vi "umgt_7thJuly2026.vi"(3 "STOP CODE":bool) -> ()   [LabVIEW 2024]
uses:
  <vilib>/DAQmx/configure/timing.llb/DAQmx Timing (Sample Clock).vi
  <vilib>/Utility/file.llb/Write Delimited Spreadsheet (string).vi
  <vilib>/Utility/file.llb/Write Delimited Spreadsheet (DBL).vi
  <vilib>/Analysis/NI_AALBase.lvlib
  <vilib>/Analysis/baseanly.llb/Mean (DBL).vi
  <vilib>/DAQmx/create/channels.llb/DAQmx Create Channel (AI-Voltage-Basic).vi
  <resource>/objmgr/daqmx.rc
  <vilib>/DAQmx/create/scale.llb/DAQmx Create Scale (Linear).vi
  <vilib>/addons/control/pid/NI_PID_pid.lvlib
  f57602c8-bb00-4a83-a2e4-247f724f5f9a.vi
  4c8e6df8-a562-4faa-a768-57c69aa10fff.vi
  3436942e-08c6-4c4c-99fa-98bd9929c734.vi
  <vilib>/Utility/error.llb/DialogType.ctl
  5b89efd5-d7eb-4bb1-b1dc-7bfe89948b2c.vi
  <vilib>/KNF LAB/Driver S/Lvlib/SIMLAB_driver_lvclass/SIMLAB_driver.lvclass
  Combustor Setup LabVIEW/Comb set up 1500W transfer from C drive/Combustor Setup LabVIEW/Bronkhorst FLOW-BUS/Bronkhorst FLOW-BUS.lvlib
  <vilib>/DAQmx/write.llb/DAQmx Write (Counter Time 1Chan 1Samp).vi
  <vilib>/DAQmx/configure/timing.llb/DAQmx Timing (Implicit).vi
  <vilib>/DAQmx/create/channels.llb/DAQmx Create Channel (CO-Pulse Generation-Time).vi
  <vilib>/DAQmx/read.llb/DAQmx Read (Analog 1D DBL NChan 1Samp).vi
  <vilib>/addons/control/pid/pid.llb/PID Advanced (DBL).vi
  <vilib>/DAQmx/read.llb/DAQmx Read (Analog 1D Wfm NChan NSamp Duration).vi
  Combustor Setup LabVIEW/Comb set up 1500W transfer from C drive/Combustor Setup LabVIEW/Bronkhorst FLOW-BUS/Public/Data/Measure/Read Measure (Direct).vi
  Combustor Setup LabVIEW/Comb set up 1500W transfer from C drive/Combustor Setup LabVIEW/Bronkhorst FLOW-BUS/Public/Data/Setpoint/Read Setpoint (Direct).vi
  <vilib>/DAQmx/read.llb/DAQmx Read (Analog 2D DBL NChan NSamp).vi
  <vilib>/KNF LAB/Driver S/Lvlib/SIMLAB_driver_lvclass/PumpAddress.ctl
  <vilib>/KNF LAB/Driver S/Lvlib/SIMLAB_driver_lvclass/InitParamCluster.ctl
  <vilib>/KNF LAB/Driver S/Lvlib/SIMLAB_driver_lvclass/PumpMode.ctl
panel:
  out "FlowRate(µL/min) out 2":i32 caption="Flow Rate (µL/min)"
  in  "Required Eq Ratio Kero":dbl min=0.0 max=1.5 step=0.01 format="%#_6f"
  out "total fuel flow":dbl
  out "p+k":dbl
  out "Bronkhorst Flow rate":dbl(graph)
  out "KNF Pump flow rate":dbl(graph)
  out "Dispensed Volume Bronkhorst":dbl(graph)
  out "Dispensed Volume KNF Pump":i32(graph)
  out "Bronkhorst Fuel Capacity Unit":string
  out "Bronkhorst Fuel Setpoint":sgl caption="Setpoint Direct"
  in  "stop 2":bool
  out "Time passed (s)":dbl
  in  "save file":bool
  out "current time":timestamp
  out "Bronkhorst Fuel Flow [g/s]":dbl format="%#_4g"
  in  "Bronkhorst Fuel [g/s]":dbl min=0.0 max=2.0 step=0.01 format="%#_4g"
  in  "GetActualVolume":bool
  out "ActualVolume(µL)":i32 caption="Actual Volume (µL)"
  in  "GetActualTime":bool
  out "Actual Time":dbl format="%<%H:%M:%S%2u>t"
  in  "GetDispenseTime":bool
  out "Dispense Time out":dbl caption="Dispense Time" format="%<%H:%M:%S%2u>t"
  in  "SetDispenseTime":bool
  in  "Dispense Time in":dbl=36000.0 caption="Dispense Time" min=1.0 max=359999.0 step=0.01 format="%<%H:%M:%S%2u>t"
  in  "GetDispenseVolume":bool
  out "DispenseVolume(µL) out":i32 caption="Dispense Volume (µL)"
  in  "SetDispenseVolume":bool
  in  "DispenseVolume(µL) in":i32 caption="Dispense Volume (µL)"
  in  "GetMode":bool
  out "Mode out":T1 caption="Mode"
  in  "GetFlowRate":bool
  out "FlowRate(µL/min) out":i32 caption="Flow Rate (µL/min)"
  in  "SetFlowRate":bool
  in  "FlowRate(µL/min) in":i32 caption="Flow Rate (µL/min)"
  in  "SetMode":bool
  in  "Mode in":T1 caption="Mode"
  in  "PrimeDrain":bool
  in  "Stop":bool
  in  "Start":bool
  in  "Pause 2":bool
  in  "Reset":bool
  in  "Close":bool
  in  "Init":bool
  in  "InitParam":T2={"VISA resource name"="COM9", "Address"=0, "UnusedLRC"=FALSE, "AckActive"=TRUE} {"Address" items=["0", "1", "2", "3", "4", "5", "6", "7", "8", "9", "10", "11", "12", "13", "14", "15", "16", "17", "18", "19", "20", "21", "22", "23", "24", "25", "26", "27", "28", "29", "30", "31", "32", "33", "34", "35", "36", "37", "38", "39", "40", "41", "42", "43", "44", "45", "46", "47", "48", "49", "50", "51", "52", "53", "54", "55", "56", "57", "58", "59", "60", "61", "62", "63", "64", "65", "66", "67", "68", "69", "70", "71", "72", "73", "74", "75", "76", "77", "78", "79", "80", "81", "82", "83", "84", "85", "86", "87", "88", "89", "90", "91", "92", "93", "94", "95", "96", "97", "98", "99"]}
  out "PumpVersion":string caption="Pump Version"
  out "FirmwareVersion":string caption="Firmware Version"
  out "error":errorcluster
  out "Status":string
  out "Near Glow plug Temperature [K]":dbl
  out "Volume units 2":bool
  in  "Volume 2":dbl=40.0 format="%.2f"
  in  "Initial Direction 2":u16(ring) items=["Infuse", "Withdraw"]
  in  "Syringe Inside Diameter (19.58 mm default)\n>14.00 mm : Volume units are mL\n<14.00 mm : Volume units are µL":dbl=28.0 min=0.1 max=50.0 step=0.01 format="%#_4g"
  in  "Pump Address (0) 2":i32 format="%0#.0f"
  in  "Baud Rate (19200) 2":u32(ring)=19200 items=["19200"=19200, "9600"=9600, "2400"=2400, "1200"=1200, "300"=300]
  in  "VISA resource name 2":refnum<visa-resource-name>="COM12"
  in  "Flow rate   2":dbl=6.0 min=0.0 max=6.0 step=0.05 format="%.3f"
  in  "Units 2":i32(ring)=2 items=["microlitters per minute (µL/min)", "microlitters per hour (µL/hr)", "milliliters per minute (mL/min)", "milliliters per hour (mL/hr)"]
  out "error out 2":errorcluster
  out "Tank 4":dbl(slide)
  out "Tank 3":dbl(slide)
  out "x+y 2":i32
  in  "RUN 2":bool
  in  "PAUSE 3":bool
  in  "PAUSE 4":bool
  out "Status 2":T4
  out "Volume Dispense 2":string
  out "Overall Eq Ratio":dbl=1.0
  in  "PID CONTROL":bool
  in  "PID SETP":dbl(slide)=20000.0 caption="speed" min=20000.0 max=200000.0 step=1000.0 scale=0.0..200000.0 scale format="%#_6p"
  in  "PID gains":T5={"proportional gain (Kc)"=0.00045, "integral time (Ti, min)"=0.15, "derivative time (Td, min)"=0.0} {"derivative time (Td, min)" format="%#.6f"; "integral time (Ti, min)" format="%#.5f"; "proportional gain (Kc)" format="%#.6f"}
  in  "Engine Type":bool=TRUE caption="1500 W"
  out "Battery %":u16 format="%_2f"
  out "error out":errorcluster
  out "full":dbl
  out "LT":dbl
  out "HT":dbl
  in  "Time to wait [ms]":u32=100
  out "DC Power [W]":dbl format="%#.1f"
  out "DC Current [A]":dbl format="%#.2f"
  out "DC Voltage [V]":dbl format="%#.2f"
  out "Ramp time":dbl format="%#.1f"
  in  "Max\nRPM":dbl=1e-05 min=1e-05 max=500000.0 step=1.0 format="%#.0f"
  in  "Ramp Up":bool
  in  "Pause":bool
  in  "Ramp Down":bool
  in  "Ramp\nRate [% sec]":dbl=0.33 min=0.0 max=1000.0 step=1.0 format="%#.2f"
  in  "STOP MOTOR":bool
  out "Shaft Speed [RPM]":dbl format="%#.0f"
  out "Atmospheric Pressure":dbl
  out "Bias Voltage":dbl
  in  "Stop - Actual":bool
  in  "Fuel Shut Off":bool
  in  "Track Fuel Flow Rate":bool
  out "Range Exceeded":bool
  out "Error Present":bool
  out "Error Text":string
  in  "Propane Flow Rate Setpoint":dbl min=0.0 max=0.3 step=0.01 format="%#_3g"
  out "Measurement Data":T6
  in  "COM Port Settings":T7={"Unit ID"="A", "Baud Rate"=enum."19200", "VISA Sesssion In"="COM13"}
  out "Bearing Temperature [degC]":dbl
  out "Generator Power":i16(graph)
  out "RPM":i32(graph)
  out "Pressure Ratio":dbl(graph)
  out "Coil Temperature":dbl(graph)
  out "Required Propane Fuel Flow Rate":dbl
  out "Equivalence Ratio propane":dbl
  in  "Required Eq Ratio Propane":dbl=0.6 min=0.0 max=1.6 step=0.1
  out "Elapsed Time":dbl
  out "Propane Fuel Flow Rate [g/s]":dbl
  out "Air Flow Rate [g/s]":dbl
  in  "Record":bool
  out "Turbine Inlet Temperature [K]":dbl
  out "Generator Coil Temperature [degC]":dbl
  out "Compressor Outlet Pressure [Pa]":dbl
  out "Inlet Pressure Delta [Pa]":dbl
  in  "Voltages":tag="cDAQ9185-1F541AEMod2/ai1, cDAQ9185-1F541AEMod2/ai5,cDAQ9185-1F541AEMod2/ai22"
  in  "Throttle %":dbl(slide)=0.001 caption="speed" min=0.001 max=100.0 step=0.1 scale=0.0..100.0
  in  "Ramping mode":u8
  # "Cal 1"
  # "Cal 2"
  # "Alicat MFC"
  # "Syringe Pump"
  # "KNF Fuel Pump"
  # "Bronkhorst Flow Controller"
  # "Totalizer Timer"
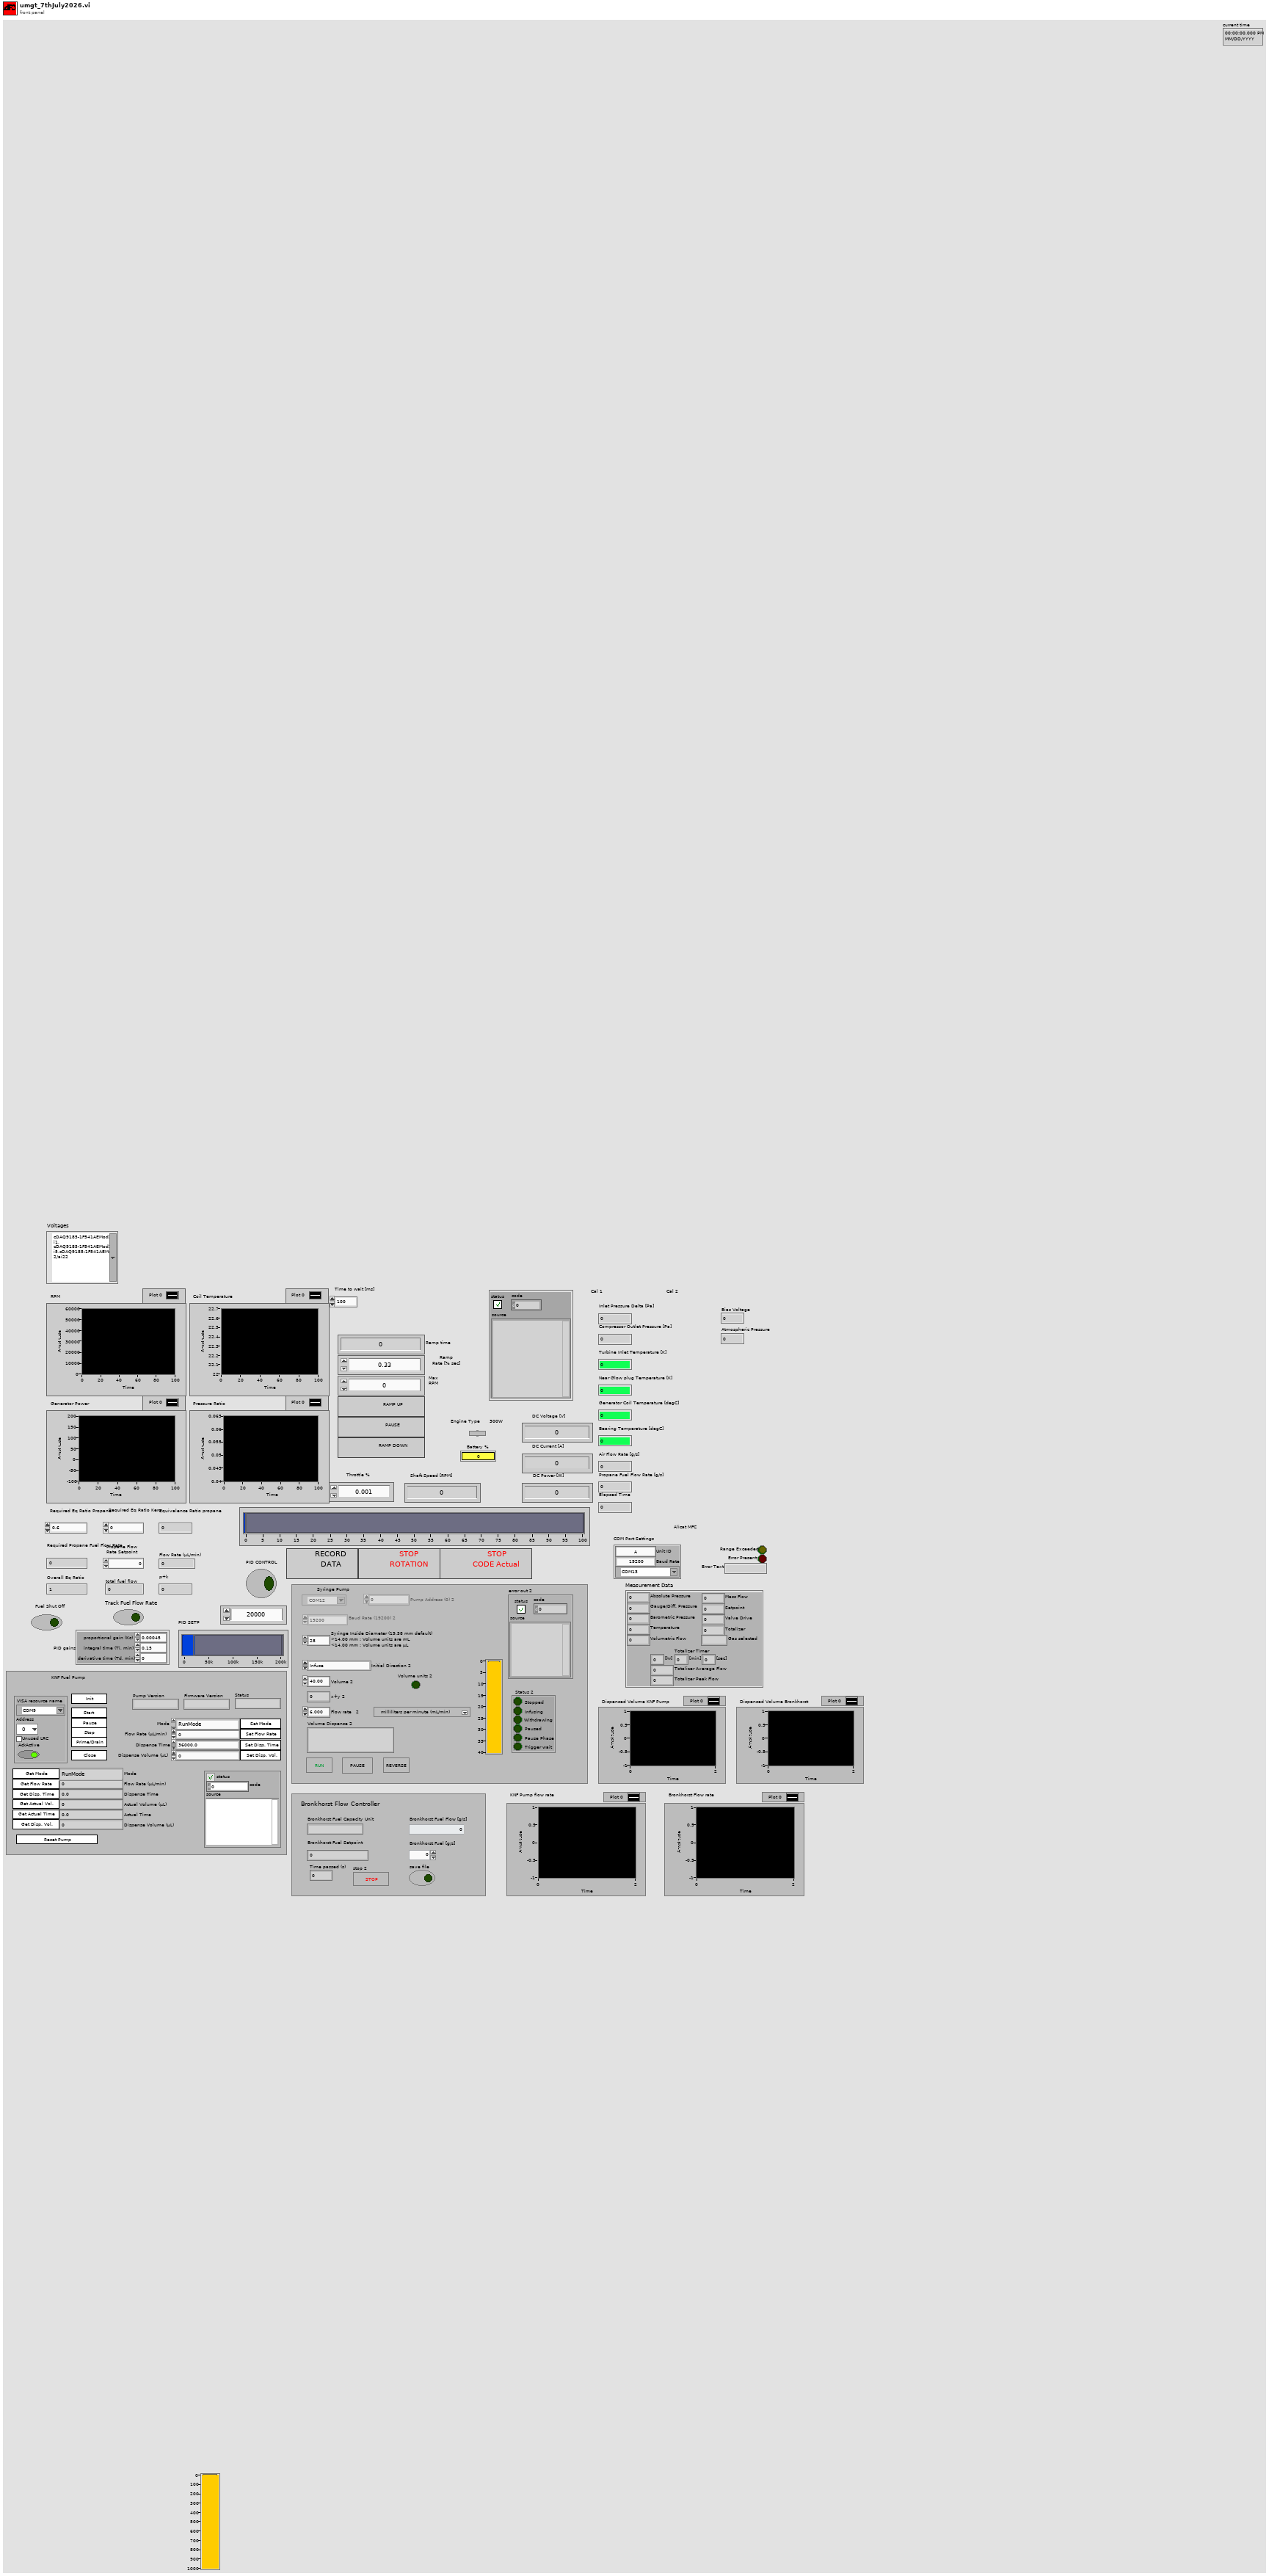
[diagram p1: front panel]
types:
  T1 = typedef "SIMLAB_driver.lvlib/SIMLAB_driver.lvclass/PumpMode.ctl" = enum16{"RunMode", "DispenseMode (mL)", "DispenseMode (mL/min)"}
  T2 = typedef "SIMLAB_driver.lvlib/SIMLAB_driver.lvclass/InitParamCluster.ctl" = cluster{"VISA resource name":refnum<visa-resource-name>, "Address":T3, "UnusedLRC":bool, "AckActive":bool}
  T3 = typedef "SIMLAB_driver.lvlib/SIMLAB_driver.lvclass/PumpAddress.ctl" = u8
  T4 = cluster{"Stopped":bool, "Infusing":bool, "Withdrawing":bool, "Paused":bool, "Pause Phase":bool, "Trigger wait":bool}
  T5 = cluster{"proportional gain (Kc)":dbl, "integral time (Ti, min)":dbl, "derivative time (Td, min)":dbl}
  T6 = cluster{"Absolute Pressure":dbl, "Gauge/Diff. Pressure":dbl, "Barometric Pressure":dbl, "Temperature":dbl, "Volumetric Flow":dbl, "Mass Flow":dbl, "Setpoint":dbl, "Valve Drive":dbl, "Totalizer":dbl, "[hr]":dbl, "[min]":dbl, "[sec]":dbl, "Totalizer Average Flow":dbl, "Totalizer Peak Flow":dbl, "Gas selected":string}
  T7 = cluster{"Unit ID":string, "Baud Rate":enum8{"2400", "9600", "19200", "38400", "57600", "115200", "Unknown"}, "VISA Sesssion In":refnum<visa-resource-name>}
  T8 = enum32{"BUS/RS232", "Analog input", "FLOW-BUS slave", "Valve close", "Controller idle", "Testing mode", "Tuning mode", "Setpoint 100%", "Valve fully open", "Calibration mode", "Analog slave", "Keyboard or FLOW-BUS setpoint", "Setpoint 0%", "FLOW-BUS analog slave", "(FPP) Range select mode", "(FPP) Manual start sensor select, automatic end sensor", "(FPP) Automatic start sensor select, manual end sensor", "(FPP) Automatic start and end sensor", "RS232 Setpoint", "RS232 broadcast mode", "Valve stearing (valve = setpoint)", "Analog valve stearing (valve = analog setpoint)", "Valve safe state"}
  T9 = typedef "DialogType.ctl" = u16
  T10 = cluster{"0=off\n1=on":u16, "Numbers of beeps\n0=continuously":dbl}
  T11 = enum8{"Enabled", "Disabled", "Disabled and Grayed Out"}
  T12 = cluster{"Absolute Pressure":bool, "Gauge/Diff. Pressure":bool, "Barometric Pressure":bool, "Temperature":bool, "Volumetric":bool, "Mass":bool, "Setpoint":bool, "Valve Drive":bool, "Totalizer":bool, "Totalizer Timer":bool, "Totalizer Average Flow":bool, "Totalizer Peak Flow":bool, "Gas Selected":bool, "Tot. Timer Format":u16}
  T13 = cluster{"Controller Full Scale":dbl, "Controller Select":u16, "Control Range":enum16{"Normal", "Inverted", "Bidirectional", "Unknown"}}
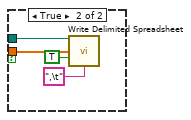
[diagram p4: hidden frame]
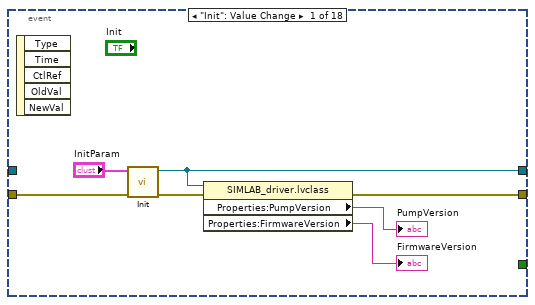
[diagram p5: hidden frame]
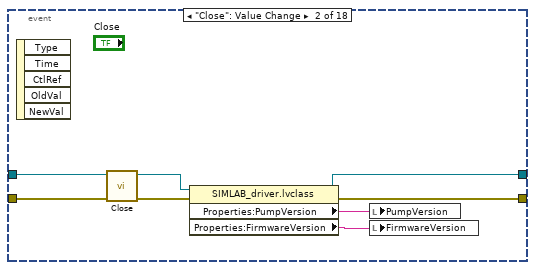
[diagram p6: hidden frame]
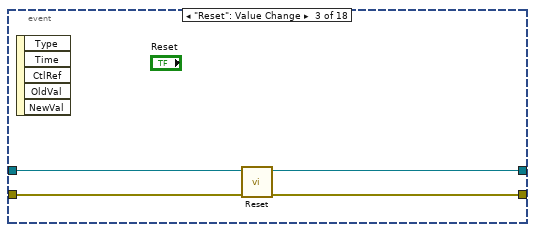
[diagram p7: hidden frame]
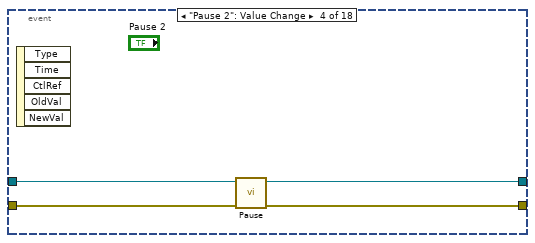
[diagram p8: hidden frame]
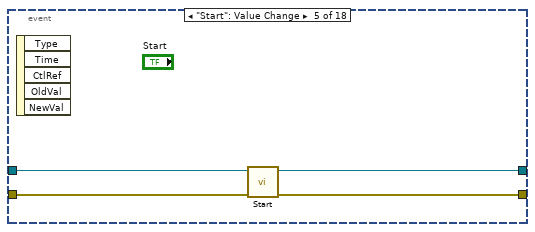
[diagram p9: hidden frame]
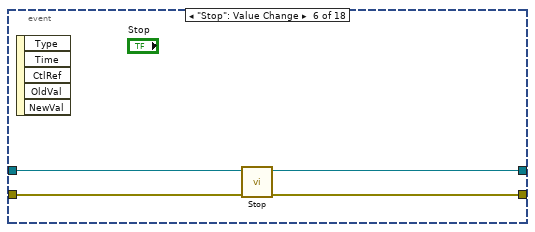
[diagram p10: hidden frame]
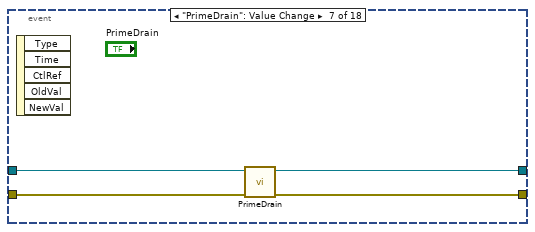
[diagram p11: hidden frame]
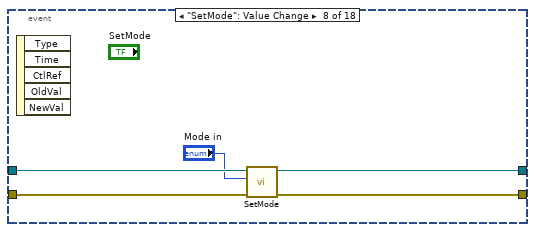
[diagram p12: hidden frame]
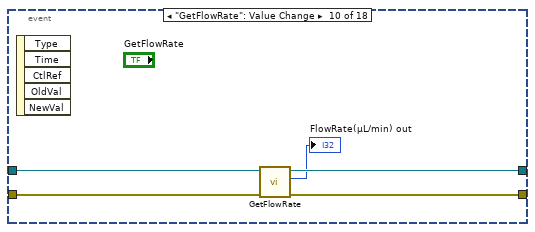
[diagram p13: hidden frame]
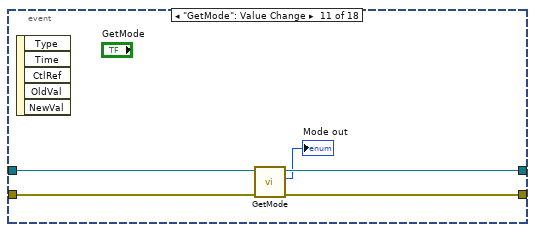
[diagram p14: hidden frame]
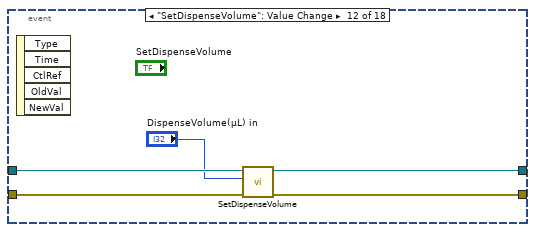
[diagram p15: hidden frame]
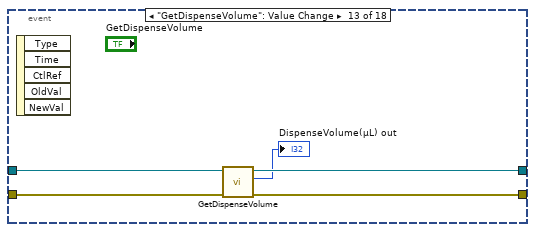
[diagram p16: hidden frame]
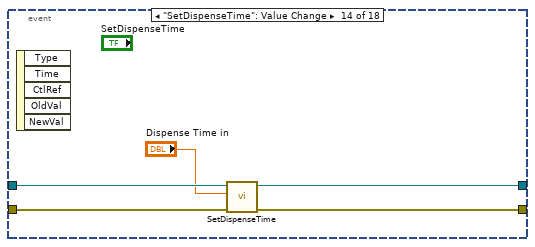
[diagram p17: hidden frame]
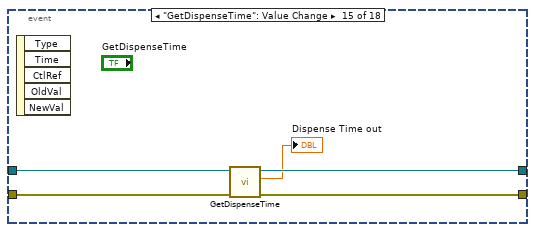
[diagram p18: hidden frame]
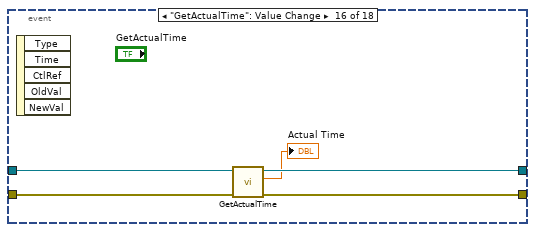
[diagram p19: hidden frame]
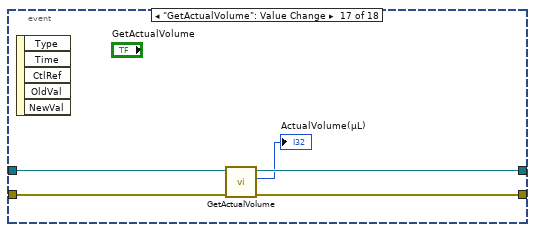
[diagram p20: hidden frame]
diagram:
  w25 = u8 3  # Node (3)
  w33 = u32 38400 items=["9600"=9600, "19200"=19200, "38400"=38400, "57600"=57600, "115200"=115200, "230400"=230400, "460800"=460800] ("Baud Rate (38400)")
  w34 = refnum<visa-resource-name> "COM5"  # VISA resource name
  w63 = T9 1 items=["no dialog", "OK message", "continue or stop message", "OK message + warnings", "continue/stop + warnings"] ("type of dialog (OK msg:1)")
  w81 = u16 0 items=["Off", "On"] ("0 = Disabled")
  # "Close the VISA session"
  # "Initialize the Com port"
  n1 = flat-sequence {
    tunnel: [w175] -> w104
    tunnel: [w174] -> w103
    tunnel: [w156] -> w102
    tunnel: [w155] -> w101
    tunnel: w104 -> [w263]
    tunnel: w103 -> [w262]
    tunnel: w102 -> [w261]
    tunnel: w101 -> [w260]
    frame #0 {
      w173 = i32[] [] ("History Data")
      n2 = Get Date/Time In Seconds() -> (seconds since 1Jan1904=w190:timestamp)
      n3 = Format Date/Time String(time format string (%c)="%y%m%d_%H_%M_%S", seconds (now)=w190) -> (date/time string=w188:string)  [unwired: 1 in]
      n4 = Concatenate Strings("D:\\UMGT Data\\Logs\\UMGT_Gen2_300W_1500W_Test_", w188, ".csv") -> (w186:string)
      n5 = Get Date/Time In Seconds() -> (seconds since 1Jan1904=w158:timestamp)
      n6 = Format Date/Time String(time format string (%c)="%y%m%d_%H_%M_%S", seconds (now)=w158) -> (date/time string=w160:string)  [unwired: 1 in]
      n7 = Concatenate Strings("D:\\UMGT Data\\Logs\\UMGT_300W_1500W_AutoLog_", w160, ".csv") -> (w162:string)
      n8 = property on="RPM" class="WFChart (strict)"("History Data"=w173) -> ()  [unwired: 2 in, 2 out]
      n9 = property on="Generator Power" class="WFChart (strict)"("History Data"=w173) -> ()  [unwired: 2 in, 2 out]
      n10 = property on="Pressure Ratio" class="WFChart (strict)"("History Data"=w173) -> ()  [unwired: 2 in, 2 out]
      n11 = property on="Coil Temperature" class="WFChart (strict)"("History Data"=w173) -> ()  [unwired: 2 in, 2 out]
      n12 = Build Array("Time [s]", "Air Flow Rate [g/s]", "Propane Fuel Flow Rate [g/s]", "Compressor Outlet Pressure [Pa]", "Coil Temperature [degC]", "Turbine Inlet Temperature [K]", "Bearing Temperature [degC]", "Controller Output Power [W]", "Shaft Speed [RPM]", "Equivalence Ratio", "Throttle %" ("element"), "Pressure Ratio" ("element"), "Overall Eq ratio" ("element"), "Inlet Pressure delta (Pa)" ("element"), "Near Glow plug Temperature (K)" ("element"), "Battery %" ("element"), "Syringe pump infuse volume" ("element"), "Syringe pump flow rate" ("element"), "KNF pump flow rate in (uL/min)" ("element"), "KNF pump flow rate out (uL/min)" ("element"), "KNF pump Dispense volume in (uL)" ("element"), "KNF pump Dispense volume out (uL)" ("element"), "KNF pump Dispense time in " ("element"), "KNF pump Dispense time out " ("element"), "Bronkhorst Fuel flow actual (g/s)" ("element"), "Bronkhorst fuel (g/s)" ("element"), "Bronkhorst Fuel set point (g/s)" ("element"), "DC Current (A)" ("element"), "DC Voltage (V)" ("element"), "Required Eq Ratio Kerosene" ("element"), "Kerosene fuel flow rate KNF (ul/min) 2 " ("element")) -> (w172:string[])
      n13 = String To Path(string=w186) -> (path=w185:path)
      n14 = String To Path(string=w162) -> (path=w163:path)
      n15 = call-poly <vilib>:"Write Delimited Spreadsheet.vi"("file path (dialog if empty)"=w163, "1D data"=w172, "delimiter (\\t)"="," ("delimiter (\\t)")) -> ("new file path (Not A Path if cancelled)"=w156:path, "error out"=w155:errorcluster)  [unwired: 11 in]
      n16 = Build Array("Time [s]", "Air Flow Rate [g/s]", "Propane Fuel Flow Rate [g/s]", "Compressor Outlet Pressure [Pa]", "Coil Temperature [degC]", "Turbine Inlet Temperature [K]", "Bearing Temperature [degC]", "Controller Output Power [W]", "Shaft Speed [RPM]", "Equivalence Ratio", "Throttle %" ("element"), "Pressure Ratio" ("element"), "Overall Eq ratio" ("element"), "Inlet Pressure Delta (Pa)" ("element"), "Near Glow plug Temperature (K)" ("element"), "Battery %" ("element"), "Syringe pump infuse volume" ("element"), "Syringe pump flow rate" ("element"), "KNF pump flow rate in (uL/min)" ("element"), "KNF pump flow rate out (uL/min)" ("element"), "KNF pump Dispense volume in (uL)" ("element"), "KNF pump Dispense volume out (uL)" ("element"), "KNF pump Dispense time in " ("element"), "KNF pump Dispense time out " ("element"), "Bronkhorst Fuel flow actual (g/s)" ("element"), "Bronkhorst fuel (g/s)" ("element"), "Bronkhorst Fuel set point (g/s)" ("element"), "DC Current (A)" ("element"), "DC Voltage (V)" ("element"), "Required Eq Ratio Kerosene" ("element"), "Kerosene fuel flow rate KNF (ul/min) 2 " ("element")) -> (w176:string[])
      n17 = call-poly <vilib>:"Write Delimited Spreadsheet.vi"("file path (dialog if empty)"=w185, "1D data"=w176, "delimiter (\\t)"="," ("delimiter (\\t)")) -> ("new file path (Not A Path if cancelled)"=w175:path, "error out"=w174:errorcluster)  [unwired: 11 in]
      "Bias Voltage" <- 0.0 ("Bias Voltage")
      "Atmospheric Pressure" <- 98600.0 ("Atmospheric Pressure")
    }
    frame #1 {
      w223 = 10106 items=["Default"=-1, "RSE"=10083, "NRSE"=10078, "Differential"=10106, "Pseudodifferential"=12529] ("input terminal configuration")
      w220 = 10123 items=["Finite Samples"=10178, "Continuous Samples"=10123, "Hardware Timed Single Point"=12522] ("sample mode")
      w214 = 10348 items=["Volts"=10348, "Amps"=10342, "Deg F"=10144, "Deg C"=10143, "Deg R"=10145, "Kelvins"=10325, "Strain"=10299, "Ohms"=10384, "Hz"=10373, "Seconds"=10364, "Meters"=10219, "Inches"=10379, "Degrees"=10146, "Radians"=10273, "Ticks"=10304, "g"=10186, "m/s^2"=12470, "m/s"=15959, "in/s"=15960, "Pascals"=10081, "Newtons"=15875, "Pounds"=15876, "kgf"=15877, "psi"=15879, "bar"=15880, "Nm"=15881, "oz-in"=15882, "lb-in"=15883, "lb-ft"=15884, "Volts/Volt"=15896, "mVolts/Volt"=15897, "pCoulombs"=16103, "Coulombs"=16102, "From TEDS"=12516] ("pre-scaled units")
      w206 = 10106 items=["Default"=-1, "RSE"=10083, "NRSE"=10078, "Differential"=10106, "Pseudodifferential"=12529] ("input terminal configuration")
      w200 = 10106 items=["Default"=-1, "RSE"=10083, "NRSE"=10078, "Differential"=10106, "Pseudodifferential"=12529] ("input terminal configuration")
      w210 = 10348 items=["Volts"=10348, "Amps"=10342, "Deg F"=10144, "Deg C"=10143, "Deg R"=10145, "Kelvins"=10325, "Strain"=10299, "Ohms"=10384, "Hz"=10373, "Seconds"=10364, "Meters"=10219, "Inches"=10379, "Degrees"=10146, "Radians"=10273, "Ticks"=10304, "g"=10186, "m/s^2"=12470, "m/s"=15959, "in/s"=15960, "Pascals"=10081, "Newtons"=15875, "Pounds"=15876, "kgf"=15877, "psi"=15879, "bar"=15880, "Nm"=15881, "oz-in"=15882, "lb-in"=15883, "lb-ft"=15884, "Volts/Volt"=15896, "mVolts/Volt"=15897, "pCoulombs"=16103, "Coulombs"=16102, "From TEDS"=12516] ("pre-scaled units")
      w203 = 10065 items=["Volts"=10348, "From Custom Scale"=10065] ("units")
      w197 = 10065 items=["Volts"=10348, "From Custom Scale"=10065] ("units")
      w192 = 10214 items=["High"=10192, "Low"=10214] ("idle state")
      w195 = 10123 items=["Finite Samples"=10178, "Continuous Samples"=10123, "Hardware Timed Single Point"=12522] ("sample mode")
      w285 = 10123 items=["Finite Samples"=10178, "Continuous Samples"=10123, "Hardware Timed Single Point"=12522] ("sample mode")
      w286 = 10123 items=["Finite Samples"=10178, "Continuous Samples"=10123, "Hardware Timed Single Point"=12522] ("sample mode")
      w291 = 10106 items=["Default"=-1, "RSE"=10083, "NRSE"=10078, "Differential"=10106, "Pseudodifferential"=12529] ("input terminal configuration")
      n18 = call-poly <vilib>:"DAQmx Create Scale.vi"("name"="SSA100-1", "slope"=80.0 ("x"), "pre-scaled units"=w210, "scaled units"="Amps") -> ("scale out"=w241:tag)  [unwired: 10 in, 1 out]
      n19 = call <vilib>:"Clear Errors.vi"() -> ("error out"=w239:errorcluster)  [unwired: 6 in, 1 out]
      n20 = call-poly <vilib>:"DAQmx Create Scale.vi"("name"="Divider", "slope"=11.0, "y-intercept"=0.0, "pre-scaled units"=w214, "scaled units"="Volts") -> ("scale out"=w240:tag)  [unwired: 9 in, 1 out]
      n21 = call-poly <vilib>:"DAQmx Create Virtual Channel.vi"("maximum value"=10.0, "minimum value"=0.0, "input terminal configuration"=w291, "physical channels"="Voltages") -> ("task out"=w288:refnum<k21>, "error out"=w287:errorcluster)  [unwired: 10 in]
      n22 = call-poly <vilib>:"DAQmx Create Virtual Channel.vi"("maximum value"=800.0, "minimum value"=-800.0, "input terminal configuration"=w200, "physical channels"=tag "cDAQ9185-1F541AEMod4/ai0", "name to assign"="MotorCurrent", "units"=w197, "error in"=w239, "custom scale name"=w241) -> ("task out"=w242:refnum<k21>, "error out"=w243:errorcluster)  [unwired: 6 in]
      n23 = call-poly <vilib>:"DAQmx Timing.vi"("task/channels in"=refnum<k21> "Near Glow Plug Temperature, Coil Temperature, Turbine Inlet Temperature, Bearing Temperature", "sample mode"=w285, "samples per channel"=1, "rate"=5.0) -> ("task out"=w278:refnum<k21>, "error out"=w277:errorcluster)  [unwired: 10 in]
      n24 = call-poly <vilib>:"DAQmx Create Virtual Channel.vi"("task in"=w242, "maximum value"=110.0, "minimum value"=-110.0, "input terminal configuration"=w206, "physical channels"=tag "cDAQ9185-1F541AEMod4/ai1", "name to assign"="MotorVoltage", "units"=w203, "error in"=w243, "custom scale name"=w240) -> ("task out"=w244:refnum<k21>, "error out"=w245:errorcluster)  [unwired: 5 in]
      n25 = call <vilib>:"Clear Errors.vi"() -> ("error out"=w238:errorcluster)  [unwired: 6 in, 1 out]
      n26 = call-poly <vilib>:"DAQmx Create Virtual Channel.vi"("task in"=w244, "maximum value"=5.0, "minimum value"=-5.0, "input terminal configuration"=w223, "physical channels"=tag "cDAQ9185-1F541AEMod4/ai2" ("counter"), "name to assign"="MotorSpeed", "error in"=w245) -> ("task out"=w246:refnum<k21>, "error out"=w247:errorcluster)  [unwired: 7 in]
      n27 = call-poly <vilib>:"DAQmx Create Virtual Channel.vi"("counter"=tag "cDAQ9185-1F541AEMod3/ctr0", "name to assign"="MotorPulse", "error in"=w238, "idle state"=w192) -> ("task out"=w234:refnum<k21>, "error out"=w235:errorcluster)  [unwired: 10 in]
      n28 = call-poly <vilib>:"DAQmx Timing.vi"("task/channels in"=w288, "sample mode"=w286, "samples per channel"=1, "rate"=150.0, "error in"=w287) -> ("task out"=w280:refnum<k21>, "error out"=w279:errorcluster)  [unwired: 9 in]
      n29 = property class="DAQmx Channel"(reference=w234, error in=w235, "CO.Pulse.Term"=tag "/cDAQ9185-1F541AEMod3/PFI0") -> (reference out=w236:refnum<k21>, error out=w237:errorcluster)
      n30 = call-poly <vilib>:"DAQmx Timing.vi"("task/channels in"=w246, "sample mode"=w220, "rate"=10000.0, "source"=tag "OnboardClock", "error in"=w247) -> ("task out"=w254:refnum<k21>, "error out"=w255:errorcluster)  [unwired: 9 in]
      n31 = call <vilib>:"DAQmx Start Task.vi"("task/channels in"=w278, "error in"=w277) -> ("task out"=w274:refnum<k21>, "error out"=w273:errorcluster)  [unwired: 12 in]
      n32 = call <vilib>:"DAQmx Start Task.vi"("task/channels in"=w280, "error in"=w279) -> ("task out"=w276:refnum<k21>, "error out"=w275:errorcluster)  [unwired: 12 in]
      n33 = call-poly <vilib>:"DAQmx Timing.vi"("task/channels in"=w236, "sample mode"=w195, "error in"=w237) -> ("task out"=w229:refnum<k21>, "error out"=w228:errorcluster)  [unwired: 11 in]
      n34 = call <vilib>:"DAQmx Start Task.vi"("task/channels in"=w254, "error in"=w255) -> ("task out"=w252:refnum<k21>, "error out"=w253:errorcluster)  [unwired: 12 in]
      n35 = call <vilib>:"High Resolution Relative Seconds.vi"() -> ("relative seconds"=w264:dbl)
      n36 = call <vilib>:"DAQmx Start Task.vi"("task/channels in"=w229, "error in"=w228) -> ("task out"=w230:refnum<k21>, "error out"=w231:errorcluster)  [unwired: 12 in]
      n37 = while {
        tunnel: w276 -> [w584]
        tunnel: w275 -> [w583]
        tunnel: w274 -> [w582]
        tunnel: w273 -> [w581]
        tunnel: [w580] -> w272
        tunnel: [w579] -> w271
        tunnel: w264 -> [w571]
        tunnel: w263 -> [w570]
        tunnel: w262 -> [w569]
        tunnel: w261 -> [w559]
        tunnel: w260 -> [w557]
        tunnel: [w508] -> w257
        tunnel: [w507] -> w256
        stop <- w578 stop-if-true
        # "change mdot from 0.702 for 1500W to 0.54 for 300W"
        # "KNF pump kerosene"
        # "changed from 15.67 to 15.5"
        # "changed from 15.67 to 15.5"
        # "ml/min to g/s\n(0.84/60)"
        # "stoichiometric propane"
        # "stoichiometric kero"
        # "Propane gas"
        # "Kerosene from syringe pump"
        n38 = call-poly <vilib>:"DAQmx Read.vi"("task/channels in"=w584, "number of samples per channel"=20, "error in"=w583) -> ("task out"=w508:refnum<k21>, "data"=w561:dbl[][], "error out"=w507:errorcluster)  [unwired: 10 in]
        n39 = Index Array(array=w561, index (row)=1 ("index")) -> (element=w547:dbl[])  [unwired: 1 in]
        n40 = Index Array(array=w561, index (row)=0 ("index")) -> (element=w548:dbl[])  [unwired: 1 in]
        n41 = call-poly <vilib>:"Mean.vi"("X"=w547) -> ("mean"=w509:dbl)  [unwired: 1 out]
        n42 = call-poly <vilib>:"Mean.vi"("X"=w548) -> ("mean"=w484:dbl)  [unwired: 1 out]
        n43 = formula code="P = 50*V;"("V"=w484) -> ("P"=w468:dbl)
        "Inlet Pressure Delta [Pa]" <- w468
        n44 = formula code="P = 16000*V;"("V"=w509) -> ("P"=w506:dbl)
        "Compressor Outlet Pressure [Pa]" <- w506
        n45 = formula code="mdot = 0.702*sqrt(Pin);"("Pin"=w468) -> ("mdot"=w566:dbl)
        "Air Flow Rate [g/s]" <- w566
        n46 = local read "Atmospheric Pressure"() -> (w513:dbl)
        n47 = local read "FlowRate(µL/min) out"() -> (w479:i32)
        n48 = local read "Measurement Data"() -> (w553:T6)
        n49 = local read "Propane Fuel Flow Rate [g/s]"() -> (w487:dbl)
        n50 = local read "Flow rate   2"() -> (w511:dbl)
        n51 = Divide(x=w506, y=w513) -> (x/y=→"Pressure Ratio":dbl)
        n52 = Multiply(x=w479, y=1.33e-05) -> (x*y=w473:dbl)
        n53 = Unbundle By Name(w553) -> ("Mass Flow"=w552:dbl)
        "Propane Fuel Flow Rate [g/s]" <- w552
        n54 = Multiply(x=w511, y=0.014) -> (x*y=w490:dbl)
        n55 = Multiply(x=15.0, y=w490) -> (x*y=w489:dbl)
        n56 = Multiply(x=15.5, y=w487) -> (x*y=w475:dbl)
        n57 = Multiply(x=15.0, y=w473) -> (x*y=w476:dbl)
        n58 = Divide(x=w566, y=w552) -> (x/y=w568:dbl)
        n59 = Multiply(x="Required Eq Ratio Propane", y=w566) -> (x*y=w564:dbl)
        n60 = Reciprocal(x=15.5) -> (1/x=w563:dbl)
        n61 = Add(x=w476, y=w475) -> (x+y=w471:dbl)
        n62 = Add(x=w489, y=w475) -> (x+y=w470:dbl)
        n63 = Divide(x=w568, y=15.5) -> (x/y=w551:dbl)
        n64 = Multiply(x=w564, y=w563) -> (x*y=→"Required Propane Fuel Flow Rate":dbl)
        n65 = Add(x=w471, y=w470) -> (x+y=w472:dbl)
        "total fuel flow" <- w472
        n66 = Reciprocal(x=w551) -> (1/x=→"Equivalence Ratio propane":dbl)
        n67 = local read "Air Flow Rate [g/s]"() -> (w486:dbl)
        n68 = Divide(x=w472, y=w486) -> (x/y=→"Overall Eq Ratio":dbl)
        n69 = disable-structure shown="Disabled" {
          frame Disabled {
            n70 = case shown="True" "Track Fuel Flow Rate" {
              frame False {
              }
              frame True {
                n71 = local read "Required Propane Fuel Flow Rate"() -> (w588:dbl)
                n72 = local read "Required Eq Ratio Kero"() -> (w587:dbl)
                n73 = Add(x=w588, y=w587) -> (x+y=w586:dbl)
                n74 = local write "Propane Flow Rate Setpoint"(w588) -> ()
                n75 = local write "p+k"(w586) -> ()
              }
            }
          }
          frame Enabled {
          }
        }
        n76 = case shown="True" "Fuel Shut Off" {
          frame False {
          }
          frame True {
            n77 = local write "Fuel Shut Off"(FALSE ("Fuel Shut Off")) -> ()
            n78 = local write "Propane Flow Rate Setpoint"(0.0 ("Fuel Flow Rate Setpoint")) -> ()
            n79 = property on="Stop" class="Bool (strict)"("Val(Sgnl)"=TRUE) -> ()  [unwired: 2 in, 2 out]
          }
        }
        n80 = local read "Dispensed Volume Bronkhorst"() -> (→"Dispensed Volume Bronkhorst":dbl)
        n81 = local read "FlowRate(µL/min) out"() -> (→"FlowRate(µL/min) out 2":i32)
        n82 = call "Elapsed Time"() -> ("Time has Elapsed"=w560:bool)  [unwired: 12 in, 7 out]
        n83 = local read "KNF Pump flow rate"() -> (→"KNF Pump flow rate":dbl)
        n84 = local read "DispenseVolume(µL) out"() -> (→"Dispensed Volume KNF Pump":i32)
        n85 = local read "Bronkhorst Flow rate"() -> (→"Bronkhorst Flow rate":dbl)
        n86 = call-poly <vilib>:"DAQmx Read.vi"("task/channels in"=w582, "error in"=w581) -> ("task out"=w580:refnum<k21>, "data"=w502:dbl[], "error out"=w579:errorcluster)  [unwired: 11 in]
        n87 = Index Array(array=w502, index=2) -> (element=w555:dbl)
        n88 = Index Array(array=w502, index=1) -> (element=w535:dbl)
        "Generator Coil Temperature [degC]" <- w535
        "Coil Temperature" <- w535
        n89 = Add(x=w555, y=273.15) -> (x+y=w515:dbl)
        "Turbine Inlet Temperature [K]" <- w515
        n90 = Index Array(array=w502, index=3) -> (element=w525:dbl)
        "Bearing Temperature [degC]" <- w525
        n91 = call <vilib>:"High Resolution Relative Seconds.vi"() -> ("relative seconds"=w572:dbl)
        n92 = Subtract(x=w572, y=w571) -> (x-y=w558:dbl)
        "Elapsed Time" <- w558
        n93 = Less Or Equal?(x=w535, y=90.0) -> (x <= y?=w540:bool)
        n94 = Greater Or Equal?(x=w535, y=50.0) -> (x >= y?=w539:bool)
        n95 = Greater?(x=w535, y=90.0) -> (0:w537:bool)
        n96 = Less?(x=w535, y=50.0) -> (x < y?=w543:bool)
        n97 = And(x=w540, y=w539) -> (x .and. y?=w538:bool)
        n98 = local read "STOP CODE"() -> (w578:bool)
        n99 = case shown="True" "Record" {
          tunnel: w558 -> [_ w681]
          tunnel: w570 -> [_ w675]
          tunnel: w569 -> [_ w674]
          frame False {
          }
          frame True {
            n100 = local read "Generator Coil Temperature [degC]"() -> (w677:dbl)
            n101 = local read "Near Glow plug Temperature [K]"() -> (w662:dbl)
            n102 = local read "Compressor Outlet Pressure [Pa]"() -> (w678:dbl)
            n103 = local read "Turbine Inlet Temperature [K]"() -> (w670:dbl)
            n104 = local read "Propane Fuel Flow Rate [g/s]"() -> (w679:dbl)
            n105 = local read "Bearing Temperature [degC]"() -> (w669:dbl)
            n106 = local read "DispenseVolume(µL) out"() -> (w655:i32)
            n107 = local read "Inlet Pressure Delta [Pa]"() -> (w663:dbl)
            n108 = local read "DispenseVolume(µL) in"() -> (w656:i32)
            n109 = local read "Equivalence Ratio propane"() -> (w667:dbl)
            n110 = local read "FlowRate(µL/min) out"() -> (w657:i32)
            n111 = local read "Bronkhorst Fuel Flow [g/s]"() -> (w652:dbl)
            n112 = local read "Bronkhorst Fuel Setpoint"() -> (w650:sgl)
            n113 = local read "FlowRate(µL/min) in"() -> (w658:i32)
            n114 = local read "Required Eq Ratio Kero"() -> (w647:dbl)
            n115 = local read "FlowRate(µL/min) out 2"() -> (w646:i32)
            n116 = local read "Shaft Speed [RPM]"() -> (w676:dbl)
            n117 = local read "Dispense Time out"() -> (w653:dbl)
            n118 = local read "Air Flow Rate [g/s]"() -> (w680:dbl)
            n119 = local read "Dispense Time in"() -> (w654:dbl)
            n120 = local read "Overall Eq Ratio"() -> (w664:dbl)
            n121 = local read "Bronkhorst Fuel [g/s]"() -> (w651:dbl)
            n122 = local read "Pressure Ratio"() -> (w665:dbl)
            n123 = local read "DC Power [W]"() -> (w671:dbl)
            n124 = local read "Flow rate   2"() -> (w659:dbl)
            n125 = local read "Throttle %"() -> (w666:dbl)
            n126 = local read "DC Current [A]"() -> (w649:dbl)
            n127 = local read "DC Voltage [V]"() -> (w648:dbl)
            n128 = local read "Battery %"() -> (w661:u16)
            n129 = local read "Tank 4"() -> (w660:dbl)
            n130 = Build Array(w681, w680, w679, w678, w677, w670, w669, w671, w676, w667, w666, w665, w664, w663, w662, w661, w660, w659, w658, w657, w656, w655, w654, w653, w652, w651, w650, w649, w648, w647, w646) -> (w672:dbl[])
            n131 = call-poly <vilib>:"Write Delimited Spreadsheet.vi"("file path (dialog if empty)"=w675, "1D data"=w672, "append to file? (new file:F)"=TRUE, "error in (no error)"=w674, "delimiter (\\t)"="," ("delimiter (\\t)")) -> ()  [unwired: 9 in, 2 out]
          }
        }
        n132 = case shown="True" w543 {
          frame False {
          }
          frame True {
            n133 = property on="Generator Coil Temperature [degC]" class="DigNum (strict)"("NumText.BGColor"=u32 1245013 ("Color Box")) -> ()  [unwired: 2 in, 2 out]
          }
        }
        n134 = case shown="False" w538 {
          frame False {
          }
          frame True {
            n135 = property on="Generator Coil Temperature [degC]" class="DigNum (strict)"("NumText.BGColor"=u32 16776770 ("Color Box")) -> ()  [unwired: 2 in, 2 out]
          }
        }
        n136 = case shown="False" w537 {
          frame False {
          }
          frame True {
            n137 = property on="Generator Coil Temperature [degC]" class="DigNum (strict)"("NumText.BGColor"=u32 16726826 ("Color Box")) -> ()  [unwired: 2 in, 2 out]
          }
        }
        n138 = Index Array(array=w502, index=0) -> (element=w503:dbl)
        n139 = case shown="True" w560 {
          tunnel: w558 -> [_ w645]
          tunnel: w559 -> [_ w638]
          tunnel: w557 -> [_ w637]
          frame False {
          }
          frame True {
            n140 = local read "Generator Coil Temperature [degC]"() -> (w641:dbl)
            n141 = local read "Overall Eq Ratio"() -> (w628:dbl)
            n142 = local read "Compressor Outlet Pressure [Pa]"() -> (w642:dbl)
            n143 = local read "Turbine Inlet Temperature [K]"() -> (w640:dbl)
            n144 = local read "Bearing Temperature [degC]"() -> (w633:dbl)
            n145 = local read "Near Glow plug Temperature [K]"() -> (w626:dbl)
            n146 = local read "Bronkhorst Fuel Flow [g/s]"() -> (w616:dbl)
            n147 = local read "Propane Fuel Flow Rate [g/s]"() -> (w643:dbl)
            n148 = local read "Bronkhorst Fuel Setpoint"() -> (w614:sgl)
            n149 = local read "Equivalence Ratio propane"() -> (w631:dbl)
            n150 = local read "Required Eq Ratio Kero"() -> (w611:dbl)
            n151 = local read "FlowRate(µL/min) out 2"() -> (w610:i32)
            n152 = local read "Inlet Pressure Delta [Pa]"() -> (w627:dbl)
            n153 = local read "Bronkhorst Fuel [g/s]"() -> (w615:dbl)
            n154 = local read "DispenseVolume(µL) out"() -> (w618:i32)
            n155 = local read "DC Power [W]"() -> (w634:dbl)
            n156 = local read "DispenseVolume(µL) in"() -> (w617:i32)
            n157 = local read "FlowRate(µL/min) out"() -> (w621:i32)
            n158 = local read "Pressure Ratio"() -> (w629:dbl)
            n159 = local read "Air Flow Rate [g/s]"() -> (w644:dbl)
            n160 = local read "Dispense Time out"() -> (w620:dbl)
            n161 = local read "Throttle %"() -> (w630:dbl)
            n162 = local read "FlowRate(µL/min) in"() -> (w622:i32)
            n163 = local read "Flow rate   2"() -> (w623:dbl)
            n164 = local read "Dispense Time in"() -> (w619:dbl)
            n165 = local read "Shaft Speed [RPM]"() -> (w639:dbl)
            n166 = local read "DC Current [A]"() -> (w613:dbl)
            n167 = local read "DC Voltage [V]"() -> (w612:dbl)
            n168 = local read "Battery %"() -> (w625:u16)
            n169 = local read "Tank 4"() -> (w624:dbl)
            n170 = Build Array(w645, w644, w643, w642, w641, w640, w633, w634, w639, w631, w630, w629, w628, w627, w626, w625, w624, w623, w622, w621, w617, w618, w619, w620, w616, w615, w614, w613, w612, w611, w610) -> (w635:dbl[])
            n171 = call-poly <vilib>:"Write Delimited Spreadsheet.vi"("file path (dialog if empty)"=w638, "1D data"=w635, "append to file? (new file:F)"=TRUE, "error in (no error)"=w637, "delimiter (\\t)"="," ("delimiter (\\t)")) -> ()  [unwired: 9 in, 2 out]
          }
        }
        n172 = Add(x=w503, y=273.15) -> (x+y=w497:dbl)
        "Near Glow plug Temperature [K]" <- w497
        n173 = Less Or Equal?(x=w525, y=90.0) -> (x <= y?=w530:bool)
        n174 = Greater Or Equal?(x=w525, y=50.0) -> (x >= y?=w531:bool)
        n175 = Greater?(x=w525, y=90.0) -> (0:w533:bool)
        n176 = Less?(x=w525, y=50.0) -> (x < y?=w527:bool)
        n177 = And(x=w530, y=w531) -> (x .and. y?=w532:bool)
        n178 = case shown="True" w527 {
          frame False {
          }
          frame True {
            n179 = property on="Bearing Temperature [degC]" class="DigNum (strict)"("NumText.BGColor"=u32 1245013 ("Color Box")) -> ()  [unwired: 2 in, 2 out]
          }
        }
        n180 = case shown="False" w532 {
          frame False {
          }
          frame True {
            n181 = property on="Bearing Temperature [degC]" class="DigNum (strict)"("NumText.BGColor"=u32 16776770 ("Color Box")) -> ()  [unwired: 2 in, 2 out]
          }
        }
        n182 = case shown="False" w533 {
          frame False {
          }
          frame True {
            n183 = property on="Bearing Temperature [degC]" class="DigNum (strict)"("NumText.BGColor"=u32 16726826 ("Color Box")) -> ()  [unwired: 2 in, 2 out]
          }
        }
        n184 = local read "Time to wait [ms]"() -> (w512:u32)
        n185 = Wait (ms)(milliseconds to wait=w512) -> ()  [unwired: 1 out]
        n186 = Less Or Equal?(x=w515, y=1050.0) -> (x <= y?=w520:bool)
        n187 = Greater Or Equal?(x=w515, y=500.0) -> (x >= y?=w519:bool)
        n188 = Greater?(x=w515, y=1050.0) -> (0:w517:bool)
        n189 = Less?(x=w515, y=500.0) -> (x < y?=w523:bool)
        n190 = And(x=w520, y=w519) -> (x .and. y?=w518:bool)
        n191 = case shown="True" w523 {
          frame False {
          }
          frame True {
            n192 = property on="Turbine Inlet Temperature [K]" class="DigNum (strict)"("NumText.BGColor"=u32 1245013 ("Color Box")) -> ()  [unwired: 2 in, 2 out]
          }
        }
        n193 = case shown="False" w518 {
          frame False {
          }
          frame True {
            n194 = property on="Turbine Inlet Temperature [K]" class="DigNum (strict)"("NumText.BGColor"=u32 16776770 ("Color Box")) -> ()  [unwired: 2 in, 2 out]
          }
        }
        n195 = case shown="False" w517 {
          frame False {
          }
          frame True {
            n196 = property on="Turbine Inlet Temperature [K]" class="DigNum (strict)"("NumText.BGColor"=u32 16726826 ("Color Box")) -> ()  [unwired: 2 in, 2 out]
          }
        }
        n197 = case shown="True" "Stop - Actual" {
          frame False {
          }
          frame True {
            n198 = local read "Shaft Speed [RPM]"() -> (w592:dbl)
            n199 = Less Or Equal?(x=w592, y=10000) -> (x <= y?=w593:bool)
            n200 = case shown="False" w593 {
              frame False {
                n201 = local write "Stop - Actual"(FALSE ("Stop - Actual")) -> ()
                n202 = One Button Dialog(message="Can't stop code while motor running") -> ()  [unwired: 1 in, 1 out]
              }
              frame True {
                n203 = local write "STOP CODE"(TRUE ("stop")) -> ()
              }
            }
          }
        }
        n204 = Less Or Equal?(x=w497, y=1050.0 ("x+y")) -> (x <= y?=w494:bool)
        n205 = Greater Or Equal?(x=w497, y=500.0) -> (x >= y?=w495:bool)
        n206 = Less?(x=w497, y=500.0) -> (x < y?=w501:bool)
        n207 = And(x=w494, y=w495) -> (x .and. y?=w500:bool)
        n208 = Greater?(x=w497, y=1050.0) -> (0:w492:bool)
        n209 = case shown="True" w501 {
          frame False {
          }
          frame True {
            n210 = property on="Near Glow plug Temperature [K]" class="DigNum (strict)"("NumText.BGColor"=u32 1245013 ("Color Box")) -> ()  [unwired: 2 in, 2 out]
          }
        }
        n211 = case shown="False" w500 {
          frame False {
          }
          frame True {
            n212 = property on="Near Glow plug Temperature [K]" class="DigNum (strict)"("NumText.BGColor"=u32 16776770 ("Color Box")) -> ()  [unwired: 2 in, 2 out]
          }
        }
        n213 = case shown="False" w492 {
          frame False {
          }
          frame True {
            n214 = property on="Near Glow plug Temperature [K]" class="DigNum (strict)"("NumText.BGColor"=u32 16726826 ("Color Box")) -> ()  [unwired: 2 in, 2 out]
          }
        }
      }
      n215 = while {
        stop <- w386 stop-if-true
        w382 = u32 100 ("millisecond multiple")
        # "15%..100%"
        n216 = Divide(x="Ramp\nRate [% sec]", y=10.0) -> (x/y=w383:dbl)
        n217 = case shown="False" "Ramp Up" {
          frame False {
          }
          frame True {
            n218 = local write "Ramping mode"(u8 1 ("Ramping mode")) -> ()
            n219 = local write "Ramp time"(0.0 ("Ramp\nTime")) -> ()
          }
        }
        n220 = case shown="False" "Ramp Down" {
          frame False {
          }
          frame True {
            n221 = local write "Ramping mode"(u8 2 ("Ramping mode")) -> ()
            n222 = local write "Ramp time"(0.0 ("Ramp\nTime")) -> ()
          }
        }
        n223 = case shown="False" "Pause" {
          frame False {
          }
          frame True {
            n224 = local write "Ramping mode"(u8 0 ("Ramping mode")) -> ()
            n225 = local write "Ramp time"(0.0 ("Ramp\nTime")) -> ()
          }
        }
        n226 = case shown="False" "STOP MOTOR" {
          frame False {
          }
          frame True {
            n227 = local write "Ramping mode"(u8 0 ("Ramping mode")) -> ()
            n228 = local write "Ramp time"(0.0 ("Ramp\nTime")) -> ()
            n229 = local write "Throttle %"(0.0 ("Ramp\nTime")) -> ()
          }
        }
        n230 = local read "Shaft Speed [RPM]"() -> (w387:dbl)
        n231 = local read "Ramping mode"() -> (w389:u8)
        n232 = local read "Engine Type"() -> (w368:bool)
        n233 = case shown="0, Default" w389 {
          tunnel: "Max\nRPM" -> [w414 _ _]
          tunnel: w387 -> [w415 _ w425]
          tunnel: w383 -> [w412 _ w422]
          tunnel: w382 -> [w409 _ w419]
          frame 0, Default {
            n234 = local read "Ramp time"() -> (w411:dbl)
            n235 = local read "Throttle %"() -> (w417:dbl)
            n236 = Greater Or Equal?(x=w415, y=w414) -> (x >= y?=w413:bool)
            n237 = case shown="False" w413 {
              frame False {
              }
              frame True {
                n238 = local write "Ramping mode"(u8 0 ("Ramping mode")) -> ()
              }
            }
            n239 = Add(x=w411, y=w409) -> (x+y=w410:dbl)
            n240 = Add(x=w417, y=w412) -> (x+y=w416:dbl)
            n241 = local write "Ramp time"(w410) -> ()
            n242 = local write "Throttle %"(w416) -> ()
          }
          frame 1 {
          }
          frame 2 {
            n243 = local read "Ramp time"() -> (w421:dbl)
            n244 = local read "Throttle %"() -> (w427:dbl)
            n245 = Less Or Equal?(x=w425, y=1000.0) -> (x <= y?=w424:bool)
            n246 = case shown="True" w424 {
              frame False {
              }
              frame True {
                n247 = local write "Ramping mode"(u8 0 ("Ramping mode")) -> ()
              }
            }
            n248 = Add(x=w421, y=w419) -> (x+y=w420:dbl)
            n249 = Subtract(x=w427, y=w422) -> (x-y=w426:dbl)
            n250 = local write "Ramp time"(w420) -> ()
            n251 = local write "Throttle %"(w426) -> ()
          }
        }
        n252 = call "Is Value Changed.vim"("value"=w368) -> ("changed or first call?"=w369:bool)
        n253 = case shown="False" w369 {
          frame False {
          }
          frame True {
            # "300w - true\n1500w - false"
            n254 = local read "Engine Type"() -> (w396:bool)
            n255 = Select(t=T5 {"proportional gain (Kc)"=0.00015, "integral time (Ti, min)"=0.075, "derivative time (Td, min)"=0.0} ("PID gains"), s=w396, f=T5 {"proportional gain (Kc)"=0.00045, "integral time (Ti, min)"=0.15, "derivative time (Td, min)"=0.0} ("PID gains")) -> (s? t:f=w395:T5)
            n256 = local write "PID gains"(w395) -> ()
          }
        }
        n257 = local read "PID CONTROL"() -> (w367:bool)
        n258 = local read "PID CONTROL"() -> (w372:bool)
        n259 = Select(t=T11."Disabled and Grayed Out" ("Disabled"), s=w367, f=T11."Enabled" ("Disabled")) -> (s? t:f=w364:T11)
        n260 = local read "STOP MOTOR"() -> (w373:bool)
        n261 = case shown="False" w372 {
          frame False {
            n262 = local read "RPM"() -> (w397:i32)
            n263 = local write "PID SETP"(w397) -> ()
          }
          frame True {
          }
        }
        n264 = case shown="False" w373 {
          frame False {
          }
          frame True {
            n265 = local write "PID CONTROL"(FALSE ("PID CONTROL")) -> ()
            n266 = local write "PID SETP"(20000.0 ("PID SETP")) -> ()
          }
        }
        n267 = local read "PID gains"() -> (w371:T5)
        n268 = property on="Throttle %" class="Slide (strict)"("DisabledEnum"=w364) -> ()  [unwired: 2 in, 2 out]
        n269 = local read "Shaft Speed [RPM]"() -> (w375:dbl)
        n270 = call "Is Value Changed.vim"("value"=w371) -> ("changed or first call?"=w370:bool)
        n271 = local read "Throttle %"() -> (w374:dbl)
        n272 = call-poly <vilib>:"PID Advanced.vi"("setpoint"="PID SETP", "output range"=cluster{"output high":dbl, "output low":dbl} {"output high"=100.0, "output low"=15.0}, "auto? (T)"="PID CONTROL", "manual control"=w374, "process variable"=w375, "PID gains"=w371, "dt (s)"=0.1, "reinitialize? (F)"=w370) -> ("output"=w377:dbl)  [unwired: 6 in, 1 out]
        n273 = local read "STOP CODE"() -> (w386:bool)
        n274 = local write "Throttle %"(w377) -> ()
        n275 = Wait Until Next ms Multiple(millisecond multiple=w382) -> ()  [unwired: 1 out]
      }
      n276 = while {
        tunnel: w252 -> [w325]
        tunnel: w253 -> [w324]
        tunnel: [w323] -> w250
        tunnel: [w322] -> w251
        stop <- w309 stop-if-true
        # "300w - true\n1500w - false"
        # "Set minimum time\nbetween loops"
        n277 = call-poly <vilib>:"DAQmx Read.vi"("task/channels in"=w325, "duration"=0.1, "error in"=w324) -> ("task out"=w323:refnum<k21>, "data"=w301:waveform(dbl)[], "error out"=w322:errorcluster)  [unwired: 10 in]
        "error out" <- w322
        n278 = Index Array(array=w301, index=0) -> (element=w304:waveform(dbl))
        n279 = Index Array(array=w301, index=1) -> (element=w300:waveform(dbl))
        n280 = Index Array(array=w301, index=2) -> (element=w299:waveform(dbl))
        n281 = call "MotorTone"("Signals"=w299) -> ("Frequency"=w311:dynamicdata)  [unwired: 9 in, 1 out]
        n282 = call "Mean(dc)"("Signals"=w304) -> ("Mean (DC)"=w321:dynamicdata)  [unwired: 13 in, 1 out]
        n283 = call "Mean(dc)3"("Signals"=w300) -> ("Mean (DC)"=w319:dynamicdata)  [unwired: 13 in, 1 out]
        n284 = local read "Throttle %"() -> (w313:dbl)
        n285 = To Double Precision Float(number=w321) -> (double precision float=w320:dbl)
        n286 = local write "DC Current [A]"(w320) -> ()
        n287 = call "Mean(dc)7"("Signals"=w311) -> ("Mean (DC)"=w310:dynamicdata)  [unwired: 13 in, 1 out]
        n288 = To Double Precision Float(number=w319) -> (double precision float=w296:dbl)
        n289 = Multiply(1:w319, 2:w321) -> (0:w308:dynamicdata)  [unwired: 1 in, 1 out]
        n290 = Greater?(x=w313, y=2.0) -> (0:w314:bool)
        n291 = To Double Precision Float(number=w308) -> (double precision float=w295:dbl)
        n292 = Select(t=60.0 ("y"), s=w314, f=0.0) -> (s? t:f=w316:dbl)
        n293 = local write "DC Voltage [V]"(w296) -> ()
        n294 = Multiply(x=w310, y=w316) -> (x*y=w318:dynamicdata)
        n295 = local read "STOP CODE"() -> (w309:bool)
        n296 = To Double Precision Float(number=w318) -> (double precision float=w307:dbl)
        n297 = local write "Generator Power"(w295) -> ()
        n298 = local write "DC Power [W]"(w295) -> ()
        n299 = local write "Shaft Speed [RPM]"(w307) -> ()
        n300 = local write "RPM"(w307) -> ()
        n301 = local read "Time to wait [ms]"() -> (w298:u32)
        n302 = Wait (ms)(milliseconds to wait=w298) -> ()  [unwired: 1 out]
        n303 = case shown="True" "Engine Type" {
          tunnel: w296 -> [w326 w350]
          tunnel: [w327 w346] -> w294
          frame False {
            # "1500w"
            # "max"
            # "min"
            n304 = Subtract(x=w326, y=39.6) -> (x-y=w339:dbl)
            n305 = Divide(x=w339, y=11.04) -> (x/y=w340:dbl)
            n306 = Multiply(x=w340, y=100.0) -> (x*y=w327:dbl)
            n307 = Greater Or Equal?(x=w327, y=25.0) -> (x >= y?=w331:bool)
            n308 = Less Or Equal?(x=w327, y=75.0) -> (x <= y?=w330:bool)
            n309 = Greater?(x=w327, y=75.0) -> (0:w328:bool)
            n310 = Less?(x=w327, y=25.0) -> (x < y?=w341:bool)
            n311 = And(x=w330, y=w331) -> (x .and. y?=w329:bool)
            n312 = case shown="False" w329 {
              frame False {
              }
              frame True {
                n313 = property on="Battery %" class="DigNum (strict)"("NumText.BGColor"=u32 16776770 ("Color Box")) -> ()  [unwired: 2 in, 2 out]
              }
            }
            n314 = case shown="True" w341 {
              frame False {
              }
              frame True {
                n315 = property on="Battery %" class="DigNum (strict)"("NumText.BGColor"=u32 16726826 ("Color Box")) -> ()  [unwired: 2 in, 2 out]
              }
            }
            n316 = case shown="False" w328 {
              frame False {
              }
              frame True {
                n317 = property on="Battery %" class="DigNum (strict)"("NumText.BGColor"=u32 1245013 ("Color Box")) -> ()  [unwired: 2 in, 2 out]
              }
            }
          }
          frame True {
            # "300w"
            n318 = Subtract(x=w350, y=18.0) -> (x-y=w358:dbl)
            n319 = Divide(x=w358, y=7.32) -> (x/y=w359:dbl)
            n320 = Multiply(x=w359, y=100.0) -> (x*y=w346:dbl)
            n321 = Greater Or Equal?(x=w346, y=25.0) -> (x >= y?=w349:bool)
            n322 = Less Or Equal?(x=w346, y=75.0) -> (x <= y?=w348:bool)
            n323 = Greater?(x=w346, y=75.0) -> (0:w345:bool)
            n324 = Less?(x=w346, y=25.0) -> (x < y?=w360:bool)
            n325 = And(x=w348, y=w349) -> (x .and. y?=w347:bool)
            n326 = case shown="False" w347 {
              frame False {
              }
              frame True {
                n327 = property on="Battery %" class="DigNum (strict)"("NumText.BGColor"=u32 16776770 ("Color Box")) -> ()  [unwired: 2 in, 2 out]
              }
            }
            n328 = case shown="True" w360 {
              frame False {
              }
              frame True {
                n329 = property on="Battery %" class="DigNum (strict)"("NumText.BGColor"=u32 16726826 ("Color Box")) -> ()  [unwired: 2 in, 2 out]
              }
            }
            n330 = case shown="False" w345 {
              frame False {
              }
              frame True {
                n331 = property on="Battery %" class="DigNum (strict)"("NumText.BGColor"=u32 1245013 ("Color Box")) -> ()  [unwired: 2 in, 2 out]
              }
            }
          }
        }
        "Battery %" <- w294
        n332 = property on="Battery %" class="DigNum (strict)"("NumText.TextColor"=u32 0) -> ()  [unwired: 2 in, 2 out]
      }
      n333 = while {
        shift-right: [w438] -> w233
        shift-left: w230 -> [w440]
        shift-right: [w437] -> w232
        shift-left: w231 -> [w439]
        shift-right: [w434] -> _
        shift-left: _ -> [w433]
        stop <- w435 stop-if-true
        # "Set minimum time\nbetween loops"
        n334 = local read "STOP MOTOR"() -> (w430:bool)
        n335 = local read "STOP CODE"() -> (w431:bool)
        n336 = local read "Throttle %"() -> (w434:dbl)
        n337 = Or(x=w431, y=w430) -> (x .or. y?=w432:bool)
        n338 = case shown="False" w432 {
          frame False {
          }
          frame True {
            # "stop values"
            n339 = local write "Throttle %"(0.001 ("Throttle M")) -> ()
          }
        }
        n340 = Not Equal?(x=w434, y=w433) -> (x != y?=w436:bool)
        n341 = case shown="False" w436 {
          tunnel: w440 -> [w443 w467]
          tunnel: w439 -> [w442 w466]
          tunnel: [w442 w465] -> w437
          tunnel: [w443 w464] -> w438
          tunnel: w434 -> [_ w456]
          frame False {
          }
          frame True {
            # "limiting to\navoid\nglitching"
            # "LT"
            # "HT"
            # "2000us\n(full with)"
            # "signal 1500..2000"
            # "% to us"
            n342 = In Range and Coerce(upper limit=100.0, x=w456, lower limit=0.0) -> (coerced(x)=w455:dbl)  [unwired: 1 out]
            n343 = Multiply(x=w455, y=5.0) -> (x*y=w462:dbl)
            n344 = Add(x=1500.0, y=w462) -> (x+y=w460:dbl)
            n345 = Multiply(x=w460, y=1e-06) -> (x*y=w446:dbl)
            "HT" <- w446
            n346 = Multiply(x=2000.0, y=1e-06) -> (x*y=w447:dbl)
            "full" <- w447
            n347 = Subtract(x=w447, y=w446) -> (x-y=w452:dbl)
            "LT" <- w452
            n348 = In Range and Coerce(upper limit=0.002, x=w446, lower limit=1e-06) -> (coerced(x)=w445:dbl)  [unwired: 1 out]
            n349 = In Range and Coerce(upper limit=0.002, x=w452, lower limit=1e-06) -> (coerced(x)=w444:dbl)  [unwired: 1 out]
            n350 = call-poly <vilib>:"DAQmx Write.vi"("task/channels in"=w467, "high time"=w445, "low time"=w444, "error in"=w466) -> ("task out"=w464:refnum<k21>, "error out"=w465:errorcluster)  [unwired: 9 in, 1 out]
          }
        }
        n351 = local read "Time to wait [ms]"() -> (w429:u32)
        n352 = Wait (ms)(milliseconds to wait=w429) -> ()  [unwired: 1 out]
        n353 = local read "STOP CODE"() -> (w435:bool)
      }
      n354 = call <vilib>:"DAQmx Stop Task.vi"("task/channels in"=w233, "error in"=w232) -> ("task out"=w226:refnum<k21>, "error out"=w227:errorcluster)  [unwired: 12 in]
      n355 = call <vilib>:"DAQmx Clear Task.vi"("task in"=w226, "error in"=w227) -> ()  [unwired: 13 in, 1 out]
      n356 = call <vilib>:"DAQmx Stop Task.vi"("task/channels in"=w250, "error in"=w251) -> ("task out"=w248:refnum<k21>, "error out"=w249:errorcluster)  [unwired: 12 in]
      n357 = call <vilib>:"DAQmx Clear Task.vi"("task in"=w248, "error in"=w249) -> ()  [unwired: 13 in, 1 out]
      n358 = call <vilib>:"DAQmx Stop Task.vi"("task/channels in"=w272, "error in"=w271) -> ("task out"=w268:refnum<k21>, "error out"=w267:errorcluster)  [unwired: 12 in]
      n359 = call <vilib>:"DAQmx Stop Task.vi"("task/channels in"=w257, "error in"=w256) -> ("task out"=w270:refnum<k21>, "error out"=w269:errorcluster)  [unwired: 12 in]
      n360 = call <vilib>:"DAQmx Clear Task.vi"("task in"=w268, "error in"=w267) -> ("error out"=w265:errorcluster)  [unwired: 13 in]
      n361 = call <vilib>:"DAQmx Clear Task.vi"("task in"=w270, "error in"=w269) -> ("error out"=w266:errorcluster)  [unwired: 13 in]
      n362 = Wait (ms)(milliseconds to wait=u32 1000) -> ()  [unwired: 1 out]
      n363 = call <vilib>:"Clear Errors.vi"("error in (no error)"=w265) -> ()  [unwired: 5 in, 2 out]
      n364 = call <vilib>:"Clear Errors.vi"("error in (no error)"=w266) -> ()  [unwired: 5 in, 2 out]
    }
    frame #2 {
      w682 = FALSE ("stop")
      n365 = local write "STOP CODE"(w682) -> ()
      n366 = local write "Stop - Actual"(w682) -> ()
    }
  }
  n367 = call "COM Port Initialization.vi"("error in (no error)"=errorcluster {"status"=FALSE, "code"=0, "source"=""}, "Communication Settings"="COM Port Settings") -> ("error out"=w41:errorcluster, "VISA Session Out"=w42:refnum<visa-resource-name>)  [unwired: 8 in]
  n368 = Unbundle By Name("COM Port Settings") -> ("Unit ID"=w40:string)
  n369 = call "Read Software Version.vi"("Unit ID (A)"=w40, "error in"=w41, "VISA Session In"=w42) -> ("error out"=w39:errorcluster, "Software Version"=w37:u8, "VISA Session Out"=w38:refnum<visa-resource-name>)  [unwired: 6 in]
  n370 = call "Read Measurement Format.vi"("Unit ID (A)"=w40, "error in"=w39, "VISA Session In"=w38) -> ("error out"=w49:errorcluster, "Data Frame Format"=w47:T12, "VISA Session Out"=w48:refnum<visa-resource-name>)  [unwired: 6 in]
  n371 = call "Read Controller Info.vi"("Unit ID (A)"=w40, "error in"=w49, "Software Version"=w37, "VISA Session In"=w48) -> ("error out"=w45:errorcluster, "Controller Info out"=w44:T13, "VISA Session Out"=w46:refnum<visa-resource-name>)  [unwired: 4 in, 1 out]
  n372 = call "NE-50X Initialize.vi"("Baud Rate (19200)"="Baud Rate (19200) 2", "VISA resource name"="VISA resource name 2") -> ("error out"=w96:errorcluster, "VISA resource name out"=w77:refnum<visa-resource-name>)  [unwired: 1 in]
  n373 = call "NE-50X Read Firmware Version.vi"("error in (no error)"=w96, "VISA resource name"=w77, "Address (0)"="Pump Address (0) 2") -> ("error out"=w95:errorcluster, "VISA resource name out"=w78:refnum<visa-resource-name>)  [unwired: 1 out]
  n374 = while {
    shift-right: [w688] -> w50
    shift-left: w45 -> [w704]
    shift-right: [w695] -> w51
    shift-left: w46 -> [w703]
    tunnel: w40 -> [w690]
    shift-right: [w692] -> _
    shift-left: w47 -> [w702]
    shift-right: [w693] -> _
    shift-left: w44 -> [w694]
    shift-right: ["Propane Flow Rate Setpoint"] -> _
    shift-left: nan ("Setpoint") -> [w691]
    shift-right: [w685] -> _
    shift-left: w37 -> [w685]
    stop <- w684 stop-if-true
    # "Write setpoint\n(if changed)"
    # "Set minimum time\nbetween loops"
    # "Acquire data"
    # "Acquire data at the requested data rate"
    n375 = call "Read Measurements.vi"("error in"=w704, "Data Frame Format In"=w702, "Unit ID (A)"=w690, "VISA Session In"=w703) -> ("error out"=w689:errorcluster, "Data Frame Format Out"=w692:T12, "Data Cluster"=→"Measurement Data":T6, "VISA Session Out"=w696:refnum<visa-resource-name>, "Unknown Dataframe Info"=w701:bool, "Error/Overrange/Unknown String"=→"Error Text":string, "Error Present"=w700:bool, "Range Exceeded"=→"Range Exceeded":bool)
    n376 = Or(x=w701, y=w700) -> (x .or. y?=→"Error Present":bool)
    n377 = local read "Time to wait [ms]"() -> (w683:u32)
    n378 = local read "STOP CODE"() -> (w684:bool)
    n379 = call "Write SetPoint.vi"("Setpoint"="Propane Flow Rate Setpoint", "Previous Setpoint"=w691, "Unit ID (A)"=w690, "error in"=w689, "Software Version"=w685, "Controller Info out"=w694, "VISA Session In"=w696) -> ("error out"=w688:errorcluster, "Controller Info out"=w693:T13, "VISA Session Out"=w695:refnum<visa-resource-name>)  [unwired: 1 in, 1 out]
    n380 = Wait (ms)(milliseconds to wait=w683) -> ()  [unwired: 1 out]
  }
  n381 = call "NE-50X Configure Alarms.vi"("error in (no error)"=w95, "Audible Alarms"=TRUE, "VISA resource name"=w78, "Address (0)"="Pump Address (0) 2") -> ("error out"=w94:errorcluster, "VISA resource name out"=w80:refnum<visa-resource-name>)
  n382 = call "NE-50X Configure Power Failure Mode.vi"("error in (no error)"=w94, "Power Failure Mode"=w81, "VISA resource name"=w80, "Address (0)"="Pump Address (0) 2") -> ("error out"=w93:errorcluster, "VISA resource name out"=w82:refnum<visa-resource-name>)
  n383 = call "NE-50X Configure Safe Mode.vi"("error in (no error)"=w93, "Safe Mode"=FALSE ("0 = Basic"), "VISA resource name"=w82, "Address (0)"="Pump Address (0) 2") -> ("error out"=w89:errorcluster, "VISA resource name out"=w83:refnum<visa-resource-name>)
  n384 = call "NE-50X Clear Volumes.vi"("error in (no error)"=w89, "VISA resource name"=w83, "Address (0)"="Pump Address (0) 2") -> ("error out"=w100:errorcluster, "VISA resource name out"=w84:refnum<visa-resource-name>)
  n385 = call "NE-50X Configure Diameter.vi"("error in (no error)"=w100, "Diameter (19.58 mm)"="Syringe Inside Diameter (19.58 mm default)\n>14.00 mm : Volume units are mL\n<14.00 mm : Volume units are µL", "VISA resource name"=w84, "Address (0)"="Pump Address (0) 2") -> ("error out"=w74:errorcluster, "Volume units"=→"Volume units 2":bool, "VISA resource name out"=w73:refnum<visa-resource-name>)
  n386 = VISA Close(VISA resource name=w51, error in (no error)=w50) -> (error out=w52:errorcluster)
  n387 = call "NE-50X Configure Volume.vi"("error in (no error)"=w74, "Volume"="Volume 2", "VISA resource name"=w73, "Address (0)"="Pump Address (0) 2") -> ("error out"=w90:errorcluster, "VISA resource name out"=w85:refnum<visa-resource-name>)
  n388 = call <vilib>:"Simple Error Handler.vi"("error in (no error)"=w52) -> ()  [unwired: 4 in, 5 out]
  n389 = call "NE-50X Configure Direction.vi"("error in (no error)"=w90, "Direction"="Initial Direction 2", "VISA resource name"=w85, "Address (0)"="Pump Address (0) 2") -> ("error out"=w91:errorcluster, "VISA resource name out"=w87:refnum<visa-resource-name>)
  n390 = call "NE-50X Buzzer.vi"("error in (no error)"=w91, "Buzzer"=T10 {"0=off\n1=on"=1, "Numbers of beeps\n0=continuously"=1.0}, "VISA resource name"=w87, "Address (0)"="Pump Address (0) 2") -> ("error out"=w62:errorcluster, "VISA resource name out"=w61:refnum<visa-resource-name>)
  n391 = while {
    shift-right: [w707] -> _
    shift-left: 0.0 -> [w706]
    stop <- w705 stop-if-true
    n392 = local read "Track Fuel Flow Rate"() -> (w708:bool)
    n393 = Wait (ms)(milliseconds to wait=u32 1000) -> ()  [unwired: 1 out]
    n394 = case shown="True" w708 {
      tunnel: [w710 w712] -> w707
      tunnel: w706 -> [w710 w713]
      frame False {
      }
      frame True {
        n395 = local read "Air Flow Rate [g/s]"() -> (w721:dbl)
        n396 = Multiply(x=w721, y="Required Eq Ratio Kero") -> (x*y=w722:dbl)
        n397 = Divide(x=w722, y=15.0) -> (x/y=w719:dbl)
        n398 = Multiply(x=w719, y=74074.0) -> (x*y=w712:dbl)
        n399 = Subtract(x=w712, y=w713) -> (x-y=w717:dbl)
        n400 = Absolute Value(x=w717) -> (abs(x)=w716:dbl)
        n401 = Greater?(x=w716, y=10.0) -> (0:w714:bool)
        n402 = case shown="True" w714 {
          tunnel: w712 -> [_ w724]
          tunnel: w713 -> [_ _]
          tunnel: w712 -> [_ _]
          frame False {
          }
          frame True {
            n403 = local write "FlowRate(µL/min) in"(w724) -> ()
            n404 = property on="SetFlowRate" class="Bool (strict)"("Val(Sgnl)"=TRUE) -> ()  [unwired: 2 in, 2 out]
          }
        }
      }
    }
    n405 = local read "Stop - Actual"() -> (w705:bool)
  }
  n406 = while {
    tunnel: w62 -> [w732]
    tunnel: w61 -> [w731]
    tunnel: "Pump Address (0) 2" -> [w730]
    tunnel: [w729] -> w59
    tunnel: [w728] -> w58
    tunnel: [w727] -> w57
    tunnel: [w726] -> w56
    tunnel: [w725] -> w55
    stop <- w784 stop-if-true
    n407 = call "Is Value Changed.vim"("value"="Flow rate   2") -> ("changed or first call?"=w734:bool)
    n408 = call "Is Value Changed.vim"("value"="Units 2") -> ("changed or first call?"=w735:bool)
    n409 = Or(x=w734, y=w735) -> (x .or. y?=w733:bool)
    n410 = case shown="False" w733 {
      tunnel: w731 -> [w786 w788]
      tunnel: w732 -> [w785 w793]
      tunnel: [w786 w792] -> w739
      tunnel: [w785 w791] -> w738
      tunnel: w730 -> [_ w787]
      tunnel: "Flow rate   2" -> [_ w790]
      tunnel: "Units 2" -> [_ w789]
      frame False {
      }
      frame True {
        n411 = call "NE-50X Configure Rate.vi"("Address (0)"=w787, "VISA resource name"=w788, "Flow"=w790, "Units"=w789, "error in (no error)"=w793) -> ("VISA resource name out"=w792:refnum<visa-resource-name>, "error out"=w791:errorcluster)
      }
    }
    n412 = call "NE-50X Query Status.vi"("error in (no error)"=w738, "VISA resource name"=w739, "Address (0)"=w730) -> ("error out"=w780:errorcluster, "Status"=w774:T4, "VISA resource name out"=w781:refnum<visa-resource-name>)
    "Status 2" <- w774
    n413 = Unbundle(w774) -> ("Infusing"=w773:bool, "Withdrawing"=w772:bool, "Paused"=w752:bool)  [unwired: 3 out]
    n414 = Or(x=w773, y=w772) -> (x .or. y?=w771:bool)
    n415 = case shown="False" w771 {
      tunnel: ["RUN 2" FALSE ("RUN")] -> w749
      frame False {
      }
      frame True {
      }
    }
    n416 = case shown="False" w749 {
      tunnel: w730 -> [w831 w832]
      tunnel: [w830 w836] -> w754
      tunnel: [w829 w835] -> w770
      tunnel: [w831 w832] -> w759
      tunnel: w781 -> [w830 w833]
      tunnel: w780 -> [w829 w834]
      frame False {
      }
      frame True {
        n417 = call "NE-50X Start Pump.vi"("error in (no error)"=w834, "VISA resource name"=w833, "Address (0)"=w832) -> ("error out"=w835:errorcluster, "VISA resource name out"=w836:refnum<visa-resource-name>)
      }
    }
    n418 = case shown="False" w749 {
      tunnel: [w800 w806] -> w751
      frame False {
        n419 = local read "x+y 2"() -> (w803:i32)
        n420 = Equal?(x=w803, y=1) -> (x = y?=w801:bool)
        n421 = case shown="False" w801 {
          tunnel: [0 1] -> w800
          frame False {
          }
          frame True {
          }
        }
      }
      frame True {
        n422 = for {
          N: 1 -> [_]
          tunnel: [w808] -> w806
          i -> [w810]
          n423 = Add(x=w810, y=1) -> (x+y=w808:i32)
          "x+y 2" <- w808
        }
      }
    }
    n424 = call "NE-50X Query Status.vi"("error in (no error)"=w770, "VISA resource name"=w754, "Address (0)"=w759) -> ("error out"=w769:errorcluster, "Status"=w762:T4, "VISA resource name out"=w768:refnum<visa-resource-name>)
    n425 = local write "Status 2"(w762) -> ()
    n426 = case shown="False" "PAUSE 4" {
      tunnel: w759 -> [w823 w824]
      tunnel: w768 -> [w821 w825]
      tunnel: w769 -> [w822 w828]
      tunnel: [w822 w827] -> w767
      tunnel: [w821 w826] -> w758
      tunnel: [w823 w824] -> w757
      frame False {
      }
      frame True {
        n427 = call "NewEraPump Stop Pump.vi"("error in (no error)"=w828, "VISA resource name"=w825, "Address (0)"=w824) -> ("error out"=w827:errorcluster, "VISA resource name out"=w826:refnum<visa-resource-name>)
      }
    }
    n428 = local read "STOP CODE"() -> (w784:bool)
    n429 = Equal?(x=w751, y=1) -> (x = y?=w725:bool)
    n430 = call "NE-50X Query Status.vi"("error in (no error)"=w767, "VISA resource name"=w758, "Address (0)"=w757) -> ("error out"=w765:errorcluster, "Status"=w761:T4, "VISA resource name out"=w766:refnum<visa-resource-name>)
    n431 = local write "Status 2"(w761) -> ()
    n432 = case shown="False" "PAUSE 3" {
      tunnel: w766 -> [w815 w816]
      tunnel: w757 -> [w813 w817]
      tunnel: [w815 w820] -> w755
      tunnel: [w814 w819] -> w764
      tunnel: w765 -> [w814 w818]
      tunnel: [w813 w817] -> w729
      frame False {
      }
      frame True {
        n433 = call "NE-50X Reverse Direction.vi"("error in (no error)"=w818, "VISA resource name"=w816, "Address (0)"=w817) -> ("error out"=w819:errorcluster, "VISA resource name out"=w820:refnum<visa-resource-name>)
      }
    }
    n434 = call "NE-50X Query Status.vi"("error in (no error)"=w764, "VISA resource name"=w755, "Address (0)"=w729) -> ("error out"=w763:errorcluster, "Status"=w760:T4, "VISA resource name out"=w756:refnum<visa-resource-name>)
    n435 = local write "Status 2"(w760) -> ()
    n436 = call "NE-50X Read Volume Dispense.vi"("error in (no error)"=w763, "VISA resource name"=w756, "Address (0)"=w729) -> ("error out"=w727:errorcluster, "Volume Dispense"=w748:string, "VISA resource name out"=w728:refnum<visa-resource-name>)
    "Volume Dispense 2" <- w748
    "error out 2" <- w727
    n437 = Fract/Exp String To Number(string=w748, offset=45) -> (number=w775:dbl)  [unwired: 2 in, 1 out]
    n438 = Fract/Exp String To Number(string=w748, offset=17) -> (offset past number=w746:i32, number=w776:dbl)  [unwired: 2 in]
    n439 = Subtract(x=w776, y=w775) -> (x-y=w741:dbl)
    n440 = Match Pattern(string=w748, regular expression=" ", offset (0)=w746) -> (after substring=w742:string)  [unwired: 3 out]
    n441 = local read "Stop - Actual"() -> (w740:bool)
    n442 = And(x=w740, y=w752) -> (x .and. y?=w726:bool)
    n443 = Match True/False String(2:"µL" ("false string"), 3:"mL" ("true string"), 4:w742) -> (0:w743:bool)  [unwired: 1 out]
    n444 = case shown="True" w743 {
      tunnel: w741 -> [w795 w797]
      frame False {
        n445 = property on="Tank 3" class="Slide (strict)"("Visible"=TRUE) -> ()  [unwired: 2 in, 2 out]
        n446 = property on="Tank 4" class="Slide (strict)"("Visible"=FALSE) -> ()  [unwired: 2 in, 2 out]
        "Tank 3" <- w795
      }
      frame True {
        n447 = property on="Tank 4" class="Slide (strict)"("Visible"=TRUE) -> ()  [unwired: 2 in, 2 out]
        n448 = property on="Tank 3" class="Slide (strict)"("Visible"=TRUE) -> ()  [unwired: 2 in, 2 out]
        "Tank 4" <- w797
      }
    }
    n449 = local read "Time to wait [ms]"() -> (w783:u32)
    n450 = Unbundle By Name(w727) -> ("status"=w753:bool)
    n451 = Compound Arithmetic op=OR(w753, w740) -> ()  [unwired: 1 out]
    n452 = Wait Until Next ms Multiple(millisecond multiple=w783) -> ()  [unwired: 1 out]
  }
  n453 = flat-sequence {
    tunnel: [errorcluster {"status"=FALSE, "code"=0, "source"=""} ("error out")] -> w36
    tunnel: [refnum<class "SIMLAB_driver.lvclass"> refnum ("SIMLAB_driver.lvlib:SIMLAB_driver.lvclass")] -> w35
    frame #0 {
      w838 = "" ("PumpVersion")
      n454 = local write "Status"(w838) -> ()
      n455 = local write "PumpVersion"(w838) -> ()
      n456 = local write "FirmwareVersion"(w838) -> ()
    }
  }
  n457 = while {
    shift-right: [w843] -> _
    shift-left: w36 -> [w849]
    shift-right: [w844] -> _
    shift-left: w35 -> [w848]
    stop <- w847 stop-if-true
    n458 = event shown="[8] \"SetFlowRate\": Value Change" {
      selector: _ -> [_ _ _ _ _ _ _ _ _ _ _ _ _ _ _ _ _ _]
      dyn-events: _ -> [_ _ _ _ _ _ _ _ _ _ _ _ _ _ _ _ _ _]
      timeout: _ -> [_ _ _ _ _ _ _ _ _ _ _ _ _ _ _ _ _ _]
      tunnel: w849 -> [w856 w864 w868 w872 w876 w880 w884 w889 w894 w899 w904 w909 w914 w919 w924 w929 w934 w937]
      tunnel: [w852 w859 w865 w870 w874 w877 w882 w886 w893 w897 w902 w906 w911 w916 w922 w927 w932 w937] -> w842
      tunnel: [_ _ _ _ _ _ _ _ _ _ _ _ _ _ _ _ _ TRUE ("Discard?")] -> w847
      tunnel: [w854 w860 w866 w869 w873 w878 w881 w887 w892 w896 w901 w907 w912 w917 w921 w926 w931 w935] -> w840
      tunnel: w848 -> [_ w863 w867 w871 w875 w879 w883 w888 w891 w898 w903 w908 w913 w918 w923 w928 w933 w935]
      event "Init": Value Change {
        n459 = event-data() -> ()  [unwired: 1 in, 5 out]
        n460 = call <vilib>:"Init.vi"("error in (no error)"=w856, "InitParam"="InitParam") -> ("error out"=w853:errorcluster, "SIMDOS out"=w854:refnum<class "SIMLAB_driver.lvclass">)  [unwired: 7 in, 1 out]
        n461 = property class="SIMLAB_driver.lvclass"(reference=w854, error in=w853) -> (error out=w852:errorcluster, "Properties:PumpVersion"=→"PumpVersion":string, "Properties:FirmwareVersion"=→"FirmwareVersion":string)  [unwired: 1 out]
      }
      event "Close": Value Change {
        n462 = event-data() -> ()  [unwired: 1 in, 5 out]
        n463 = call <vilib>:"Close.vi"("error in (no error)"=w864, "SIMDOS in"=w863) -> ("error out"=w862:errorcluster, "SIMDOS out"=w861:refnum<class "SIMLAB_driver.lvclass">)  [unwired: 8 in]
        n464 = property class="SIMLAB_driver.lvclass"(reference=w861, error in=w862) -> (reference out=w860:refnum<class "SIMLAB_driver.lvclass">, error out=w859:errorcluster, "Properties:PumpVersion"=w858:string, "Properties:FirmwareVersion"=w857:string)
        n465 = local write "PumpVersion"(w858) -> ()
        n466 = local write "FirmwareVersion"(w857) -> ()
      }
      event "Reset": Value Change {
        n467 = event-data() -> ()  [unwired: 1 in, 5 out]
        n468 = call <vilib>:"Reset.vi"("error in (no error)"=w868, "SIMDOS in"=w867) -> ("error out"=w865:errorcluster, "SIMDOS out"=w866:refnum<class "SIMLAB_driver.lvclass">)  [unwired: 8 in]
      }
      event "Pause 2": Value Change {
        n469 = event-data() -> ()  [unwired: 1 in, 5 out]
        n470 = call <vilib>:"Pause.vi"("error in (no error)"=w872, "SIMDOS in"=w871) -> ("error out"=w870:errorcluster, "SIMDOS out"=w869:refnum<class "SIMLAB_driver.lvclass">)  [unwired: 8 in]
      }
      event "Start": Value Change {
        n471 = event-data() -> ()  [unwired: 1 in, 5 out]
        n472 = call <vilib>:"Start.vi"("error in (no error)"=w876, "SIMDOS in"=w875) -> ("error out"=w874:errorcluster, "SIMDOS out"=w873:refnum<class "SIMLAB_driver.lvclass">)  [unwired: 8 in]
      }
      event "Stop": Value Change {
        n473 = event-data() -> ()  [unwired: 1 in, 5 out]
        n474 = call <vilib>:"Stop.vi"("error in (no error)"=w880, "SIMDOS in"=w879) -> ("error out"=w877:errorcluster, "SIMDOS out"=w878:refnum<class "SIMLAB_driver.lvclass">)  [unwired: 8 in]
      }
      event "PrimeDrain": Value Change {
        n475 = event-data() -> ()  [unwired: 1 in, 5 out]
        n476 = call <vilib>:"PrimeDrain.vi"("error in (no error)"=w884, "SIMDOS in"=w883) -> ("error out"=w882:errorcluster, "SIMDOS out"=w881:refnum<class "SIMLAB_driver.lvclass">)  [unwired: 8 in]
      }
      event "SetMode": Value Change {
        n477 = event-data() -> ()  [unwired: 1 in, 5 out]
        n478 = call <vilib>:"SetMode.vi"("error in (no error)"=w889, "Mode"="Mode in", "SIMDOS in"=w888) -> ("error out"=w886:errorcluster, "SIMDOS out"=w887:refnum<class "SIMLAB_driver.lvclass">)  [unwired: 7 in]
      }
      event "SetFlowRate": Value Change {
        n479 = event-data() -> ()  [unwired: 1 in, 5 out]
        n480 = call <vilib>:"SetFlowRate.vi"("error in (no error)"=w894, "FlowRate"="FlowRate(µL/min) in", "SIMDOS in"=w891) -> ("error out"=w893:errorcluster, "SIMDOS out"=w892:refnum<class "SIMLAB_driver.lvclass">)  [unwired: 7 in]
      }
      event "GetFlowRate": Value Change {
        n481 = event-data() -> ()  [unwired: 1 in, 5 out]
        n482 = call <vilib>:"GetFlowRate.vi"("error in (no error)"=w899, "SIMDOS in"=w898) -> ("error out"=w897:errorcluster, "FlowRate"=→"FlowRate(µL/min) out":i32, "SIMDOS out"=w896:refnum<class "SIMLAB_driver.lvclass">)  [unwired: 7 in]
      }
      event "GetMode": Value Change {
        n483 = event-data() -> ()  [unwired: 1 in, 5 out]
        n484 = call <vilib>:"GetMode.vi"("error in (no error)"=w904, "SIMDOS in"=w903) -> ("error out"=w902:errorcluster, "Mode"=→"Mode out":T1, "SIMDOS out"=w901:refnum<class "SIMLAB_driver.lvclass">)  [unwired: 7 in]
      }
      event "SetDispenseVolume": Value Change {
        n485 = event-data() -> ()  [unwired: 1 in, 5 out]
        n486 = call <vilib>:"SetDispenseVolume.vi"("error in (no error)"=w909, "DispenseVolume"="DispenseVolume(µL) in", "SIMDOS in"=w908) -> ("error out"=w906:errorcluster, "SIMDOS out"=w907:refnum<class "SIMLAB_driver.lvclass">)  [unwired: 7 in]
      }
      event "GetDispenseVolume": Value Change {
        n487 = event-data() -> ()  [unwired: 1 in, 5 out]
        n488 = call <vilib>:"GetDispenseVolume.vi"("error in (no error)"=w914, "SIMDOS in"=w913) -> ("error out"=w911:errorcluster, "DispenseVolume"=→"DispenseVolume(µL) out":i32, "SIMDOS out"=w912:refnum<class "SIMLAB_driver.lvclass">)  [unwired: 7 in]
      }
      event "SetDispenseTime": Value Change {
        n489 = event-data() -> ()  [unwired: 1 in, 5 out]
        n490 = call <vilib>:"SetDispenseTime.vi"("error in (no error)"=w919, "DispenseTime"="Dispense Time in", "SIMDOS in"=w918) -> ("error out"=w916:errorcluster, "SIMDOS out"=w917:refnum<class "SIMLAB_driver.lvclass">)  [unwired: 7 in]
      }
      event "GetDispenseTime": Value Change {
        n491 = event-data() -> ()  [unwired: 1 in, 5 out]
        n492 = call <vilib>:"GetDispenseTime.vi"("error in (no error)"=w924, "SIMDOS in"=w923) -> ("error out"=w922:errorcluster, "DispenseTime"=→"Dispense Time out":dbl, "SIMDOS out"=w921:refnum<class "SIMLAB_driver.lvclass">)  [unwired: 7 in]
      }
      event "GetActualTime": Value Change {
        n493 = event-data() -> ()  [unwired: 1 in, 5 out]
        n494 = call <vilib>:"GetActualTime.vi"("error in (no error)"=w929, "SIMDOS in"=w928) -> ("error out"=w927:errorcluster, "ActualTime"=→"Actual Time":dbl, "SIMDOS out"=w926:refnum<class "SIMLAB_driver.lvclass">)  [unwired: 7 in]
      }
      event "GetActualVolume": Value Change {
        n495 = event-data() -> ()  [unwired: 1 in, 5 out]
        n496 = call <vilib>:"GetActualVolume.vi"("error in (no error)"=w934, "SIMDOS in"=w933) -> ("error out"=w932:errorcluster, "ActualVolume"=→"ActualVolume(µL)":i32, "SIMDOS out"=w931:refnum<class "SIMLAB_driver.lvclass">)  [unwired: 7 in]
      }
      event Panel Close? {
        n497 = event-data() -> ()  [unwired: 1 in, 3 out]
        n498 = event-data("Discard?"=TRUE) -> ()  [unwired: 1 in, 1 out]
      }
    }
    "error" <- w842
    n499 = call <vilib>:"Simple Error Handler.vi"("error in (no error)"=w842) -> ("error out"=w846:errorcluster)  [unwired: 4 in, 4 out]
    n500 = call <vilib>:"Clear Errors.vi"("error in (no error)"=w846) -> ("error out"=w841:errorcluster)  [unwired: 5 in, 1 out]
    n501 = property class="SIMLAB_driver.lvclass"(reference=w840, error in=w841) -> (reference out=w844:refnum<class "SIMLAB_driver.lvclass">, error out=w843:errorcluster, "Properties:Status"=→"Status":string)
  }
  n502 = Format Date/Time String(time format string (%c)="%d.%m.%Y_%H.%M.%S") -> (date/time string=w14:string)  [unwired: 2 in]
  n503 = call "Initialize.vi"("Baud Rate (38400)"=w33, "Node (3)"=w25, "VISA resource name"=w34) -> ("error out"=w32:errorcluster, "VISA resource name out"=w31:refnum<visa-resource-name>)  [unwired: 7 in]
  n504 = Concatenate Strings("FlowController_" ("string"), w14, ".csv" ("string")) -> (w10:string)
  n505 = Build Array("Time passed (sec)", "Timestamp" ("element"), "Initial Fuel flow rate setpoint (g/s)" ("element"), "Flow rate fuel (g/s)" ("element"), "Final Fuel flow rate setpoint (g/s)" ("element")) -> (w6:string[])
  n506 = call "Wink.vi"("error in (no error)"=w32, "Node (3)"=w25, "VISA resource name"=w31) -> ("error out"=w28:errorcluster, "VISA resource name out"=w30:refnum<visa-resource-name>)  [unwired: 7 in]
  n507 = Build Path(base path=path "D:/UMGT Data/Logs/Bronkhorst flow controller logs", name or relative path=w10) -> (appended path=w12:path)
  n508 = call <vilib>:"High Resolution Relative Seconds.vi"() -> ("relative seconds"=w9:dbl)
  n509 = call-poly <vilib>:"Write Delimited Spreadsheet.vi"("file path (dialog if empty)"=w12, "1D data"=w6, "delimiter (\\t)"=",\t" ("delimiter (\\t)")) -> ("new file path (Not A Path if cancelled)"=w8:path)  [unwired: 11 in, 1 out]
  n510 = call "Configure Control Mode.vi"("error in (no error)"=w28, "Control Mode (0: BUS/RS232)"=T8."BUS/RS232", "Node (3)"=w25, "VISA resource name"=w30) -> ("error out"=w27:errorcluster, "VISA resource name out"=w29:refnum<visa-resource-name>)  [unwired: 6 in]
  n511 = while {
    shift-right: [w957] -> w23
    shift-left: w27 -> [w965]
    shift-right: [w956] -> w24
    shift-left: w29 -> [w964]
    shift-right: [w955] -> w20
    shift-left: w25 -> [w955]
    tunnel: w9 -> [w951]
    tunnel: w8 -> [w946]
    stop <- "stop 2" stop-if-true
    # "Bronkhorst Fuel Flow Controller"
    n512 = local read "Bronkhorst Fuel [g/s]"() -> (w943:dbl)
    n513 = call <vilib>:"High Resolution Relative Seconds.vi"() -> ("relative seconds"=w952:dbl)
    n514 = call "Read Capacity Unit.vi"("error in (no error)"=w965, "Node (3)"=w955, "VISA resource name"=w964) -> ("error out"=w963:errorcluster, "Capacity Unit"=→"Bronkhorst Fuel Capacity Unit":string, "VISA resource name out"=w962:refnum<visa-resource-name>)  [unwired: 6 in]
    n515 = Get Date/Time In Seconds() -> (seconds since 1Jan1904=w942:timestamp)
    "current time" <- w942
    n516 = Format Date/Time String(time format string (%c)="%H:%M:%S", seconds (now)=w942) -> (date/time string=w940:string)  [unwired: 1 in]
    n517 = Subtract(x=w952, y=w951) -> (x-y=w950:dbl)
    "Time passed (s)" <- w950
    n518 = call "Configure Setpoint (Direct).vi"("error in (no error)"=w963, "Setpoint Direct (0)"=w943, "Node (3)"=w955, "VISA resource name"=w962) -> ("error out"=w961:errorcluster, "VISA resource name out"=w960:refnum<visa-resource-name>)  [unwired: 6 in]
    n519 = Decimal String To Number(string=w940) -> (number=w939:i32)  [unwired: 2 in, 1 out]
    n520 = call-poly "Read Measure.vi"("error in (no error)"=w961, "Node (3)"=w955, "VISA resource name"=w960) -> ("error out"=w958:errorcluster, "Measure Direct"=w944:sgl, "VISA resource name out"=w959:refnum<visa-resource-name>)  [unwired: 6 in]
    n521 = local write "Bronkhorst Fuel Flow [g/s]"(w944) -> ()
    n522 = call-poly "Read Setpoint.vi"("error in (no error)"=w958, "Node (3)"=w955, "VISA resource name"=w959) -> ("error out"=w957:errorcluster, "Setpoint Direct"=w945:sgl, "VISA resource name out"=w956:refnum<visa-resource-name>)  [unwired: 6 in]
    "Bronkhorst Fuel Setpoint" <- w945
    n523 = Build Array(w950, w939, w943, w944, w945) -> (w947:dbl[])
    n524 = case shown="False" "save file" {
      tunnel: w947 -> [_ w967]
      tunnel: w946 -> [_ w966]
      frame False {
      }
      frame True {
        n525 = call-poly <vilib>:"Write Delimited Spreadsheet.vi"("file path (dialog if empty)"=w966, "1D data"=w967, "append to file? (new file:F)"=TRUE, "delimiter (\\t)"=",\t" ("delimiter (\\t)")) -> ()  [unwired: 10 in, 2 out]
      }
    }
    n526 = Wait Until Next ms Multiple(millisecond multiple=u32 100) -> ()  [unwired: 1 out]
  }
  n527 = case shown="False" w55 {
    tunnel: [w970 w982] -> w71
    tunnel: w57 -> [w970 w981]
    tunnel: w58 -> [w971 w980]
    tunnel: w59 -> [w972 w979]
    tunnel: [w971 w978] -> w67
    tunnel: [w972 w977] -> w65
    tunnel: w56 -> [_ w973]
    frame False {
    }
    frame True {
      n528 = call "NewEraPump Stop Pump.vi"("error in (no error)"=w981, "VISA resource name"=w980, "Address (0)"=w979) -> ("error out"=w976:errorcluster, "VISA resource name out"=w975:refnum<visa-resource-name>)
      n529 = local write "x+y 2"(0 ("x+y")) -> ()
      n530 = case shown="True" w973 {
        tunnel: w976 -> [w987 w990]
        tunnel: [w986 w990] -> w982
        tunnel: w979 -> [w983 w988]
        tunnel: [w985 w989] -> w978
        tunnel: w975 -> [w984 w989]
        tunnel: [w983 w988] -> w977
        frame False {
          n531 = call "NewEraPump Stop Pump.vi"("error in (no error)"=w987, "VISA resource name"=w984, "Address (0)"=w983) -> ("error out"=w986:errorcluster, "VISA resource name out"=w985:refnum<visa-resource-name>)
        }
        frame True {
        }
      }
    }
  }
  n532 = call "NE-50X Query Status.vi"("error in (no error)"=w71, "VISA resource name"=w67, "Address (0)"=w65) -> ("error out"=w69:errorcluster, "Status"=w68:T4, "VISA resource name out"=w70:refnum<visa-resource-name>)
  n533 = local write "Status 2"(w68) -> ()
  n534 = call "NE-50X Reset Pump.vi"("error in (no error)"=w69, "VISA resource name"=w70) -> ("error out"=w66:errorcluster, "VISA resource name out"=w72:refnum<visa-resource-name>)
  n535 = call "NE-50X Close.vi"("VISA resource name"=w72, "error in (no error)"=w66) -> ("error out"=w64:errorcluster)  [unwired: 13 in]
  n536 = call <vilib>:"General Error Handler.vi"("type of dialog (OK msg:1)"=w63, "error in (no error)"=w64) -> ()  [unwired: 9 in, 5 out]
  n537 = call "Configure Control Mode.vi"("error in (no error)"=w23, "Control Mode (0: BUS/RS232)"=T8."BUS/RS232", "Node (3)"=w20, "VISA resource name"=w24) -> ("error out"=w21:errorcluster, "VISA resource name out"=w22:refnum<visa-resource-name>)  [unwired: 6 in]
  n538 = call <vilib>:"Close.vi"("error in (no error)"=w21, "VISA resource name"=w22) -> ("error out"=w18:errorcluster)  [unwired: 9 in]
  n539 = call <vilib>:"Simple Error Handler.vi"("error in (no error)"=w18) -> ()  [unwired: 4 in, 5 out]
